vi "Main_FPGA_1_2.vi"() -> ()   [LabVIEW 2018]
uses:
  <vilib>/FPGAPlugInAG/NI 9148/niLvFpga_Open_NI 9148.vi
  <vilib>/rvi/interface/common/dynamic/niFpgaDynamicAddResources.vi
  <vilib>/FPGAPlugInAG/Dynamic/niLvFpga_Reset_Dynamic.vi
  <vilib>/FPGAPlugInAG/Dynamic/niLvFpga_Run_Dynamic.vi
  <vilib>/FPGAPlugInAG/cRIO-9082/niLvFpga_Open_cRIO-9082.vi
  <vilib>/addons/control/pid/pid.llb/PID (DBL).vi
  <vilib>/rvi/errors/niLvFpgaAdjustHostInterfaceError.vi
  <vilib>/FPGAPlugInAG/Dynamic/niLvFpga_Abort_Dynamic.vi
  <vilib>/FPGAPlugInAG/Dynamic/niLvFpga_Close_Dynamic.vi
  <vilib>/Utility/file.llb/Write Delimited Spreadsheet (string).vi
  <vilib>/rvi/interface/nirviOpenFPGA/nirviOpenFPGA.xnode
  FPGA Bitfiles/Expansion chassis.lvbitx
  Main_Mess_FPGA.vi
  <vilib>/rvi/interface/nirviMethod/nirviMethod.xnode
  FPGA Bitfiles/Main_FPGA_V3.lvbitx
  Main_FPGA.vi
  <vilib>/rvi/interface/nirviReadWriteControl/nirviReadWriteControl.xnode
  <vilib>/rvi/interface/nirviCloseFPGA/nirviCloseFPGA.xnode
  <vilib>/rvi/interface/Simulation/niFpgaSimulationCallBeginRW.vi
  <vilib>/addons/control/pid/NI_PID_pid.lvlib
  NiFpgaLv.dll
panel:
  in  "File Nmae":string
  out "Engine_Limits":refnum<vi>[](array[refnum])
  out "Pressure_Limits":refnum<vi>[](array[refnum])
  out "Pressure_Sensors":refnum<vi>[](array[refnum])
  out "Temp_Limits":refnum<vi>[](array[refnum])
  out "error out":errorcluster
  in  "Config_Save":bool
  out "Config File":path
  in  "Power_Max_Lim":dbl=100.0
  in  "Oil_P":T1={"Gain"=1.0, "offset"=0.0}
  in  "Exhaust_P":T1={"Gain"=0.5, "offset"=0.0}
  in  "Coolant-Out_P":T1={"Gain"=0.5, "offset"=0.0}
  in  "Coolant-In_P":T1={"Gain"=0.5, "offset"=0.0}
  in  "Intercooler-In_P":T1={"Gain"=1.0, "offset"=0.0}
  in  "Intercooler-Out_P":T1={"Gain"=1.0, "offset"=0.0}
  in  "Misc_P":T1={"Gain"=1.0, "offset"=0.0}
  in  "Misc_P_Lim":fxp<+/-,48,10>=5.0
  in  "Intercooler-Out_P_Lim":fxp<+/-,48,10>=3.0
  in  "Intercooler-In_P_Lim":fxp<+/-,48,10>=3.0
  in  "Intercooler_Out_Temp_lim":dbl=60.0 format="%#_13g"
  out "Intercooler_Out_T":dbl(knob) scale=0.0..100.0 scale format="%3d"
  out "Boolean 7":bool
  in  "Speed_Max_Lim":dbl=8000.0
  in  "Torque_Min_Lim":dbl=-1000.0
  in  "Torque_Max_Lim":dbl=1000.0
  out "AI0":dbl
  out "AI1":dbl
  out "AI2":dbl
  out "Mod1/CH0":fxp<+/-,32,7>
  out "Mod1/CH1":fxp<+/-,32,7>
  out "Mod1/CH2":fxp<+/-,32,7>
  out "Mod1/CH3":fxp<+/-,32,7>
  out "Intercooler-Out_P":dbl(slide) scale=0.0..10.0 scale format="%#1_6g"
  out "Misc_P":dbl(slide) scale=0.0..10.0 scale format="%#1_6g"
  out "Intercooler_In_T":dbl(knob) scale=0.0..100.0 scale format="%3d"
  out "Boolean":bool
  out "Boolean 2":bool
  out "Exhaust_T":dbl(knob) scale=0.0..1000.0 scale format="%3d"
  out "Oil_T":dbl(knob) scale=0.0..140.0 scale format="%3d"
  out "Boolean 3":bool
  out "Coolant_Outlet_T":dbl(knob) scale=0.0..120.0 scale format="%3d"
  out "Boolean 5":bool
  out "Coolant_Inlet_T":dbl(knob) scale=0.0..120.0 scale format="%3d"
  out "Boolean 4":bool
  out "Basement_T":dbl(knob) scale=0.0..60.0 scale format="%3d"
  out "Boolean 6":bool
  out "Speed Summary":dbl(knob) scale=0.0..8000.0
  out "Torque Summary":dbl(knob) scale=-500.0..1000.0
  out "Power":dbl(knob) scale=0.0..300.0
  out "Oil_P":dbl(slide) scale=0.0..10.0 scale format="%#1.1g"
  out "Exhaust_P":dbl(slide) scale=0.0..5.0 scale format="%#1_6g"
  out "Coolant-Out_P":dbl(slide) scale=0.0..5.0
  out "Intercooler-In_P":dbl(slide) scale=0.0..10.0 scale format="%2d"
  out "Coolant-In_P":dbl(slide) scale=0.0..5.0
  in  "Data_Log":bool
  in  "Coolant_Inlet_Temp_Lim":dbl=95.0 format="%#_13g"
  in  "Oil_Pres_Max_lim":fxp<+/-,48,10>=7.0
  in  "Exhaust_Pres_Lim":fxp<+/-,48,10>=3.0
  in  "CoolantOut_press_Lim":fxp<+/-,48,10>=3.0
  in  "Intercooler_In_Temp_lim":dbl=90.0 format="%#_13g"
  in  "Exhaust_Temp_Lim":dbl=730.0 format="%#_13g"
  in  "Coolant_Outlet_Temp_Lim":dbl=100.0 format="%#_13g"
  in  "Coolant In Pres_Lim":fxp<+/-,48,10>=3.0
  in  "Oil_Temp_Max_Lim":dbl=120.0 format="%#_13g"
  in  "Oil_Temp_min_Lim":dbl=20.0 format="%#_13g"
  in  "Oil_Pres_Min_lim":fxp<+/-,48,10>=1.0
  out "Saftey_Lim_error":bool
  in  "Ambient_pressure":fxp<+/-,48,10>=0.9399999999986903
  in  "Basement_Temp_Lim":dbl=2000.0 format="%#_13g"
  in  "Pres_min_spd_lim":dbl=800.0
  out "Waveform Chart - Dark":cluster{"Numeric":dbl, "Numeric":dbl}(graph)
  out "Temperature out":dbl
  in  "PID gains":T2={"proportional gain (Kc)"=1.0, "integral time (Ti, min)"=0.1, "derivative time (Td, min)"=0.0} {"derivative time (Td, min)" format="%.3f"; "integral time (Ti, min)" format="%.3f"; "proportional gain (Kc)" format="%.3f"}
  in  "Output range":cluster{"Output high":dbl, "Output low":dbl}={"Output high"=10.0, "Output low"=0.0} {"Output low" format="%.2f"; "Output high" format="%.2f"}
  in  "Temperature PID":bool=TRUE
  in  "Temperature":dbl(slide) scale=0.0..100.0
  in  "Stop":bool
  # "Engine Safety Limits"
  # "Pressure Safety Limits"
  # "Temp Safety Limits"
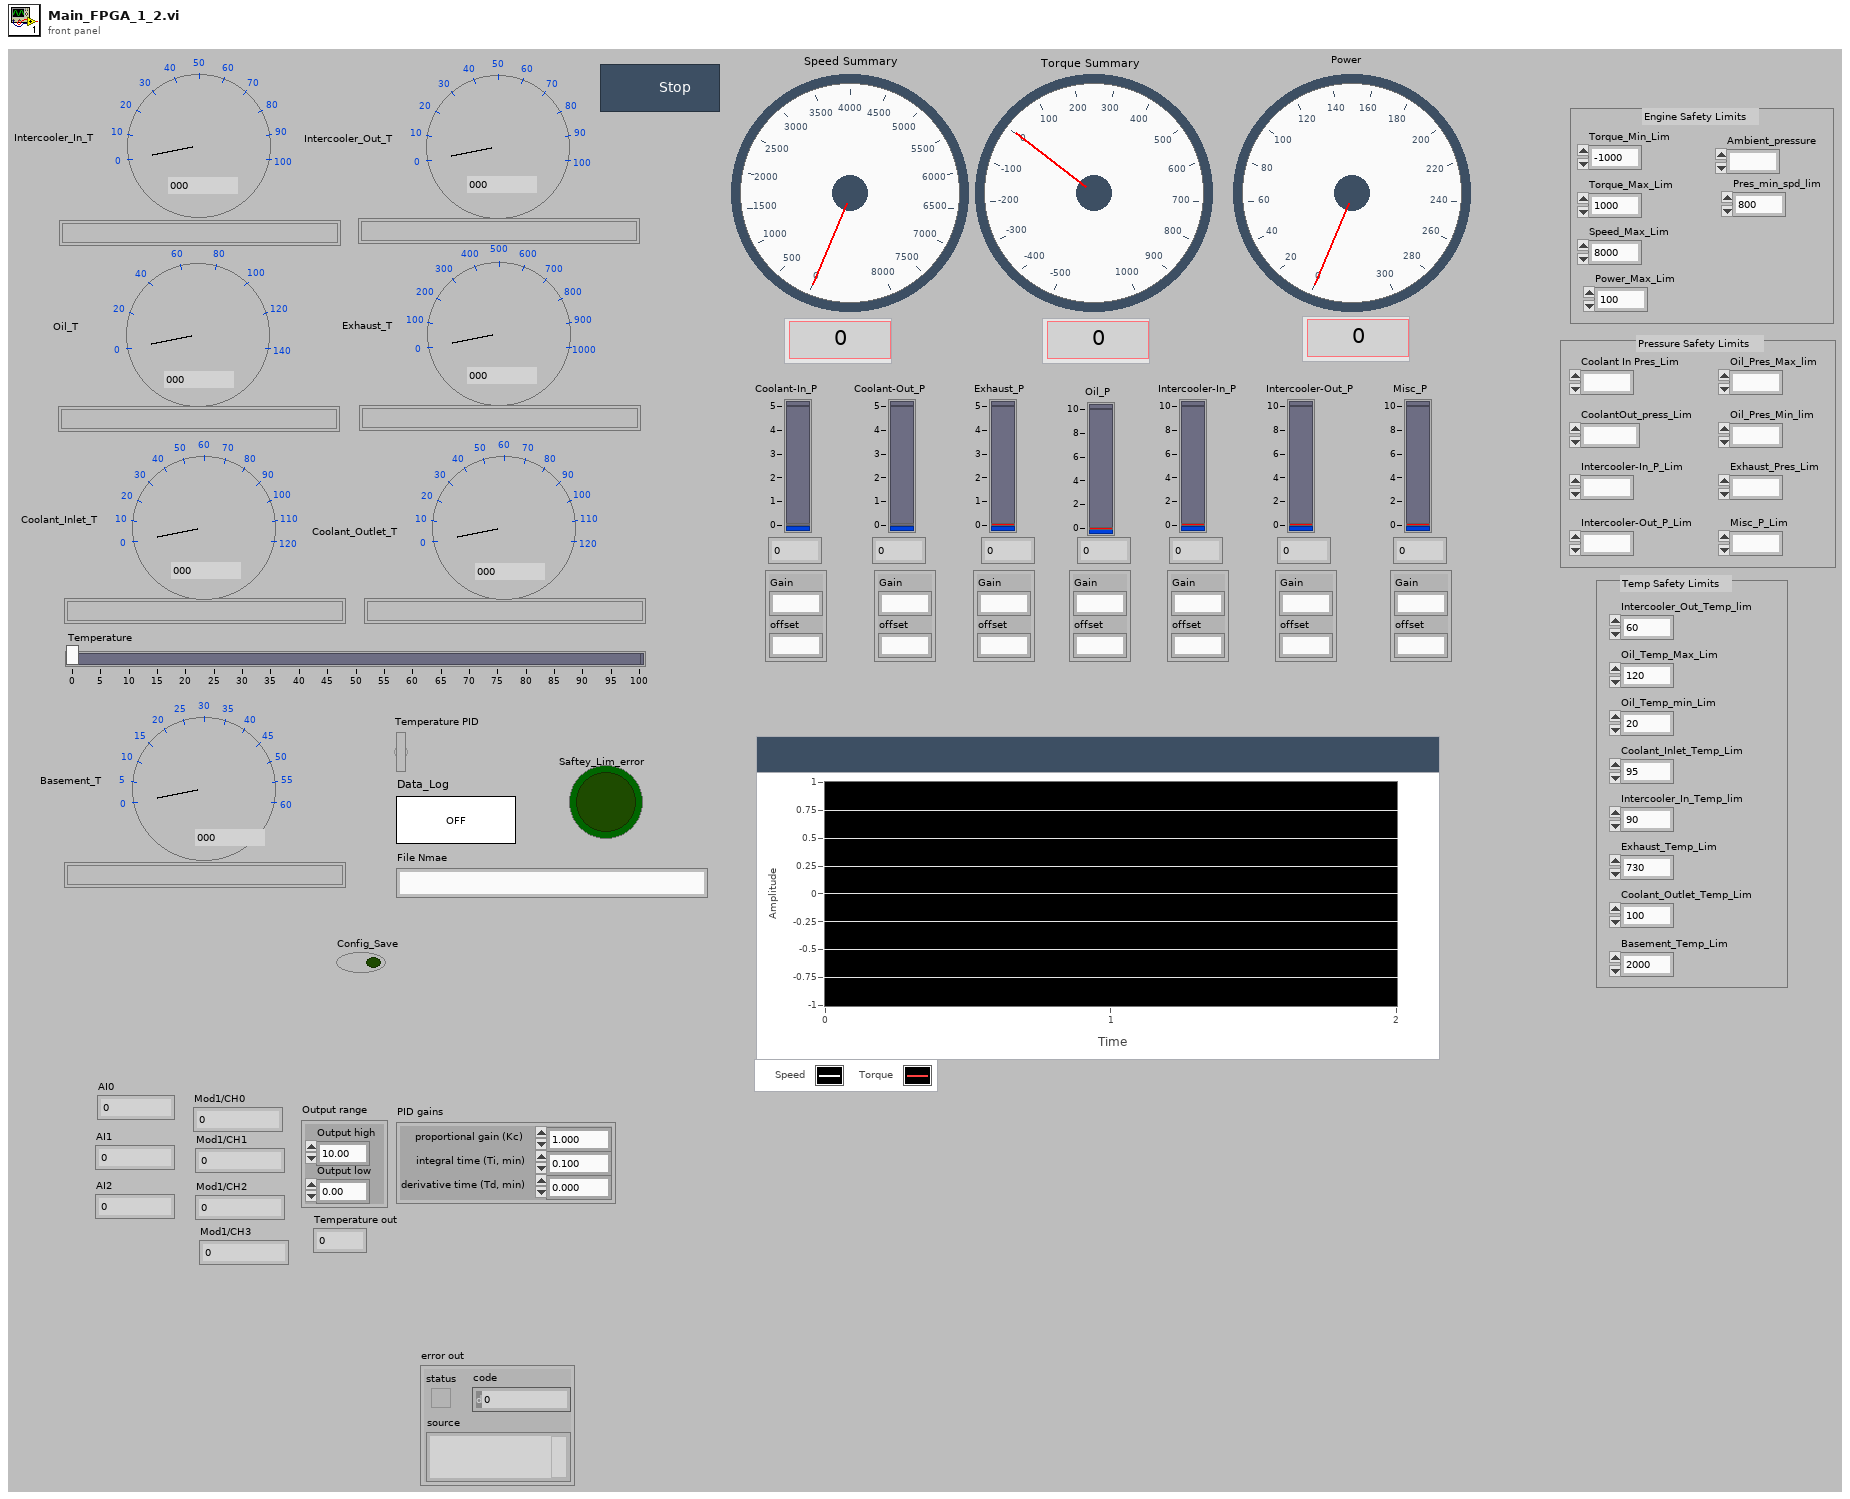
[diagram p1: front panel]
types:
  T1 = cluster{"Gain":fxp<+/-,24,5>, "offset":fxp<+/-,24,5>}
  T2 = cluster{"proportional gain (Kc)":dbl, "integral time (Ti, min)":dbl, "derivative time (Td, min)":dbl}
  T3 = enum32{"Invalid", "Standard", "Closed", "Hidden", "Minimized", "Maximized"}
  T4 = enum32{"invalid app kind", "Development System", "Run Time System", "Student Edition", "Embedded LabVIEW", "Evaluation", "Custom"}
  T5 = cluster{"Core":cluster{"Current VI Reference":refnum<vi>, "Close Panel on Exit?":bool}, "Intercooler_In_T":refnum<vi>, "Coolant_Inlet_T":refnum<vi>, "Coolant_Outlet_T":refnum<vi>, "Basement_T":refnum<vi>, "Exhaust_T":refnum<vi>, "Oil_T":refnum<vi>, "Intercooler_Out_T":refnum<vi>, "ExpansionChassFPGA":refnum<k20>}
  T6 = cluster{"Current VI Reference":refnum<vi>, "Close Panel on Exit?":bool}
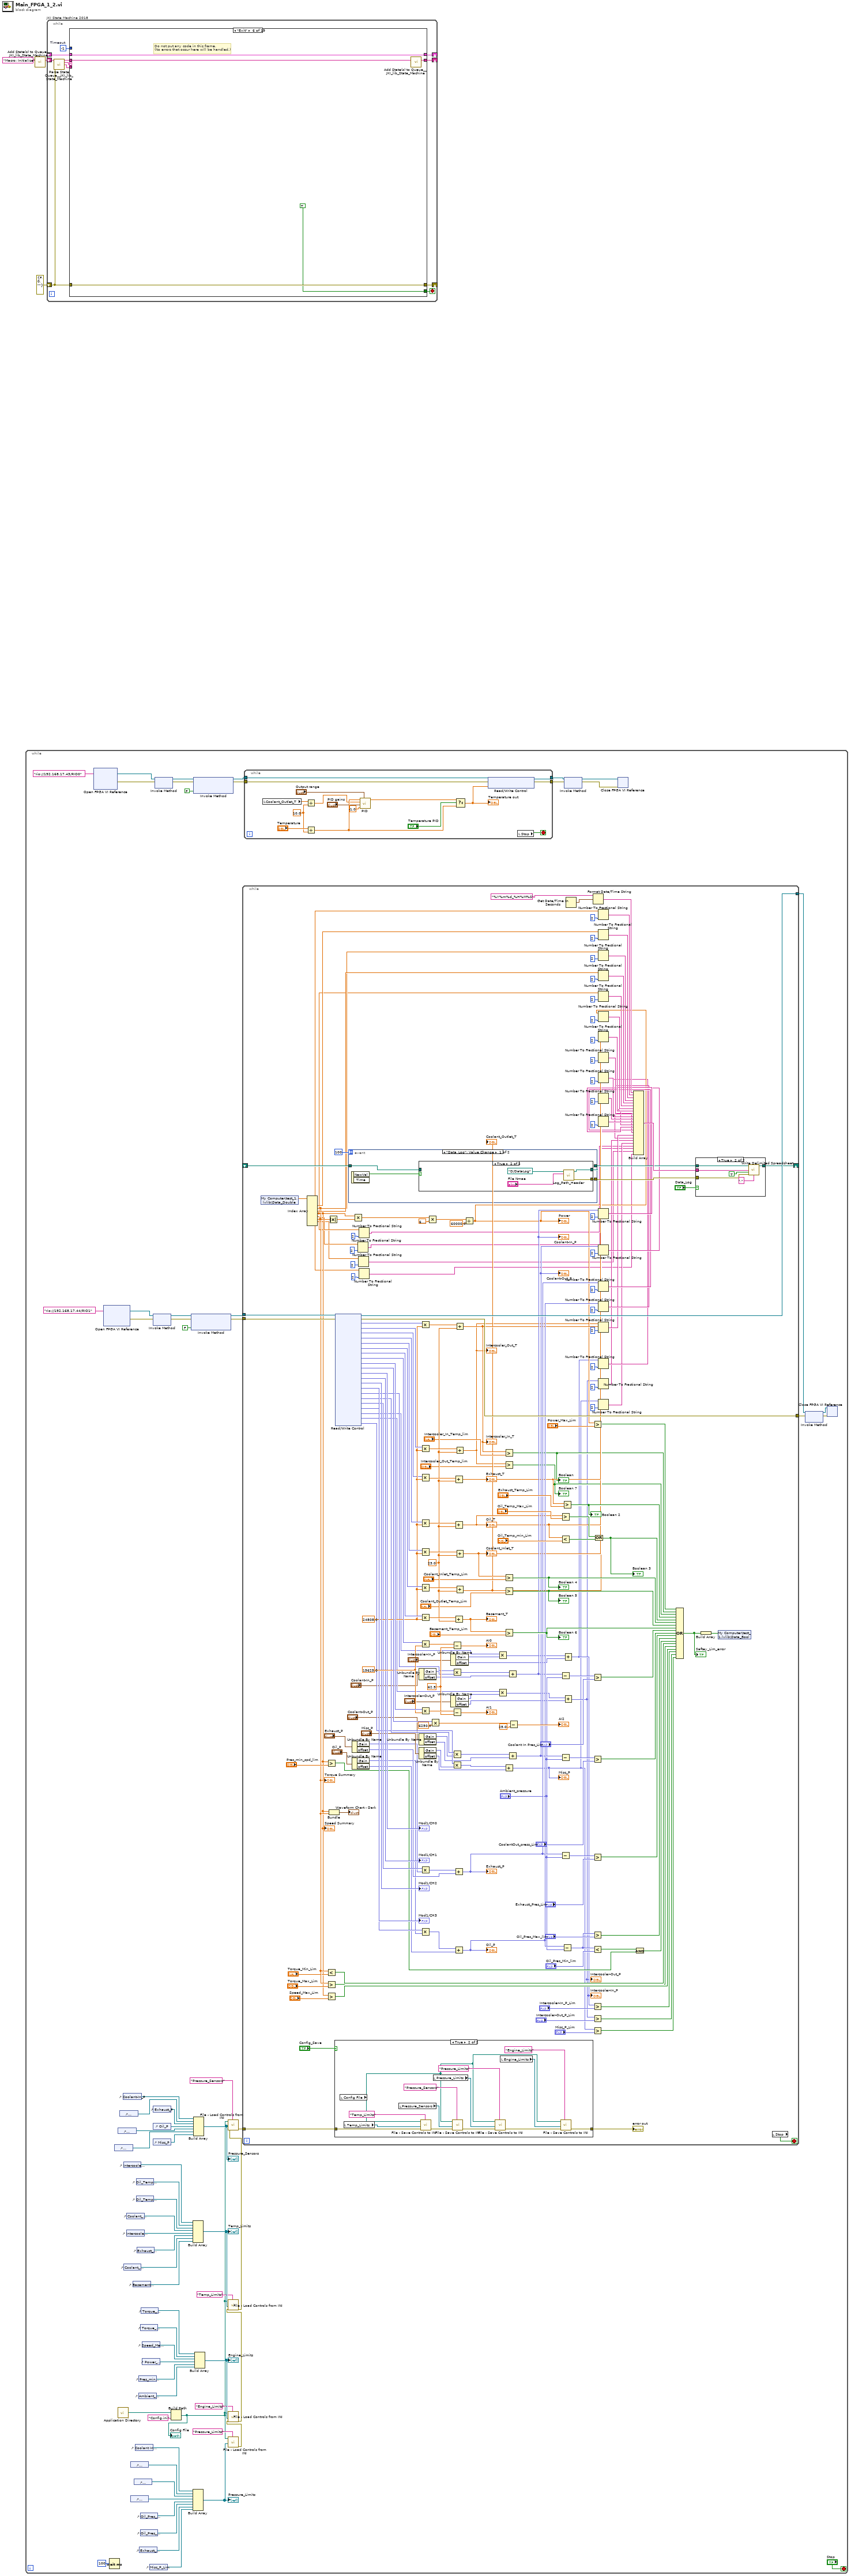
[diagram p0: block diagram]
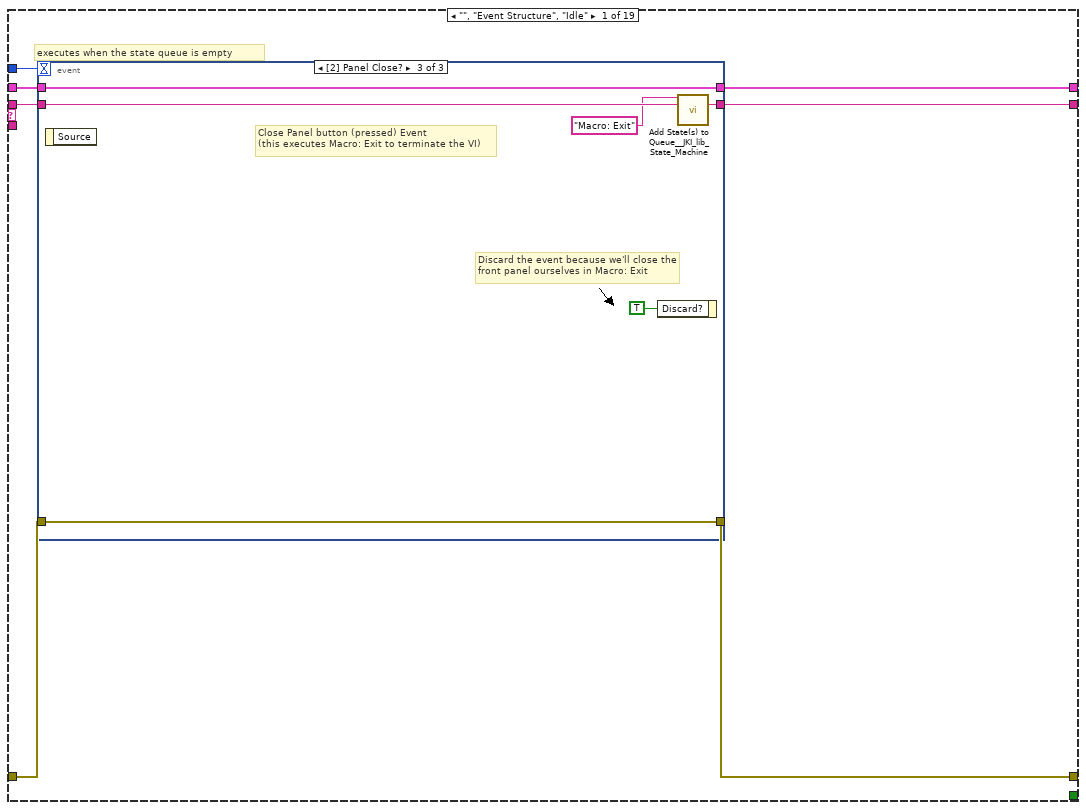
[diagram p2: hidden frame]
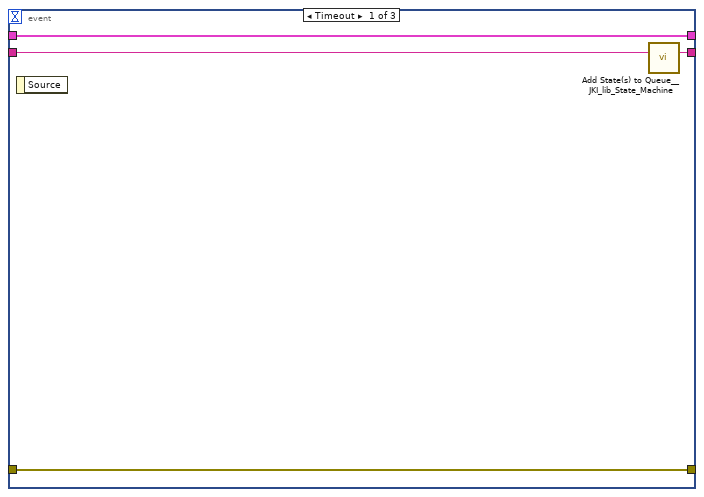
[diagram p3: hidden frame]
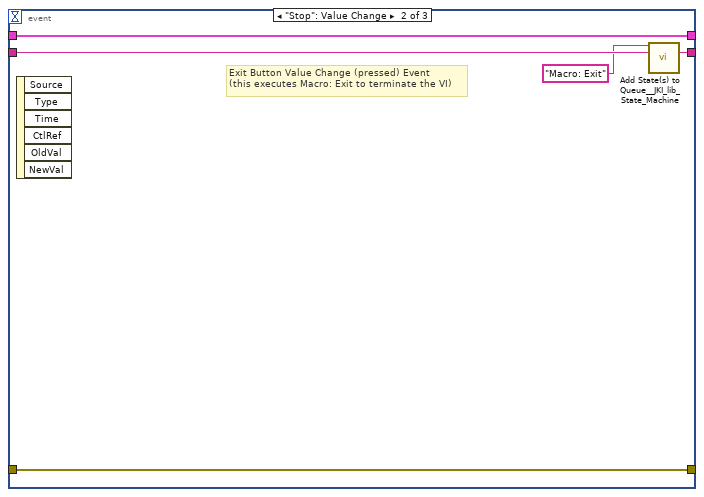
[diagram p4: hidden frame]
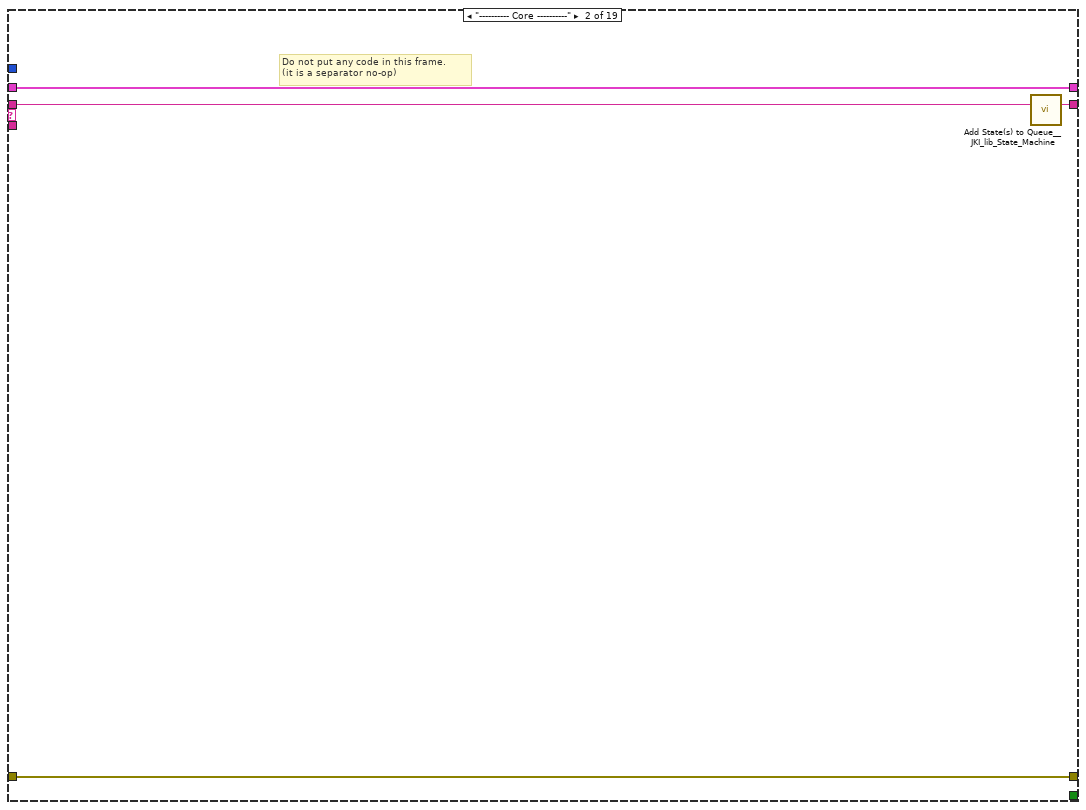
[diagram p5: hidden frame]
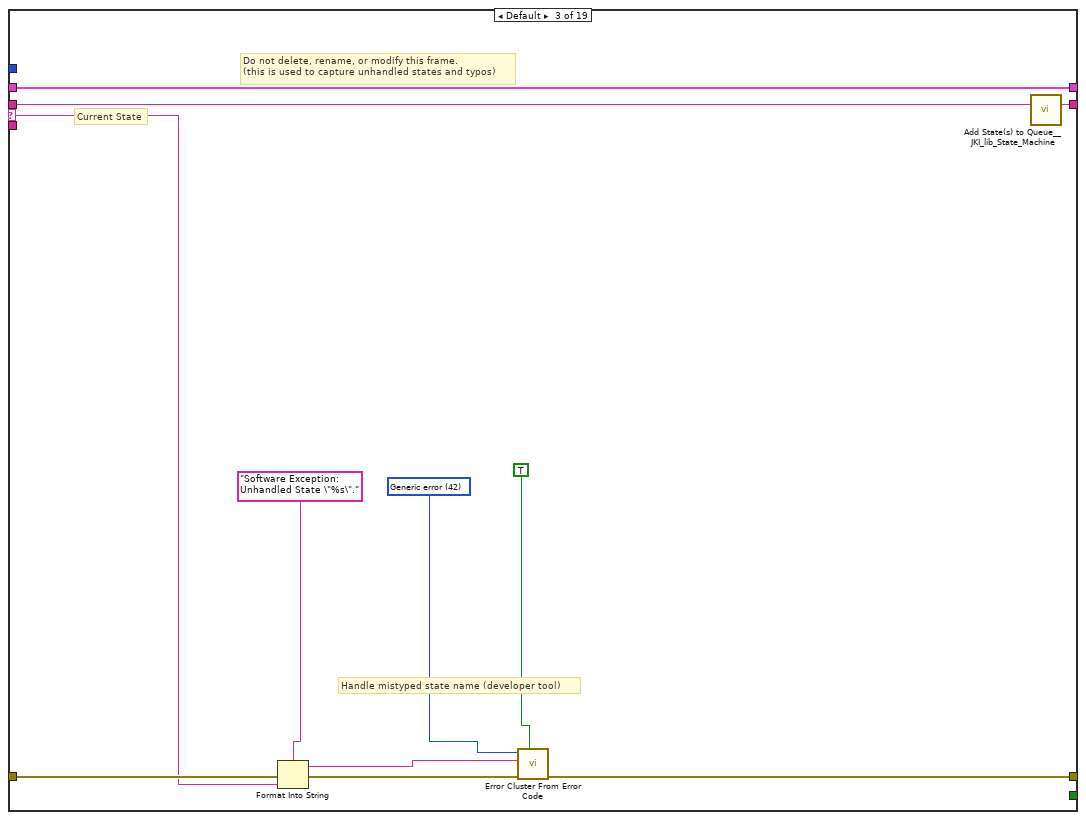
[diagram p6: hidden frame]
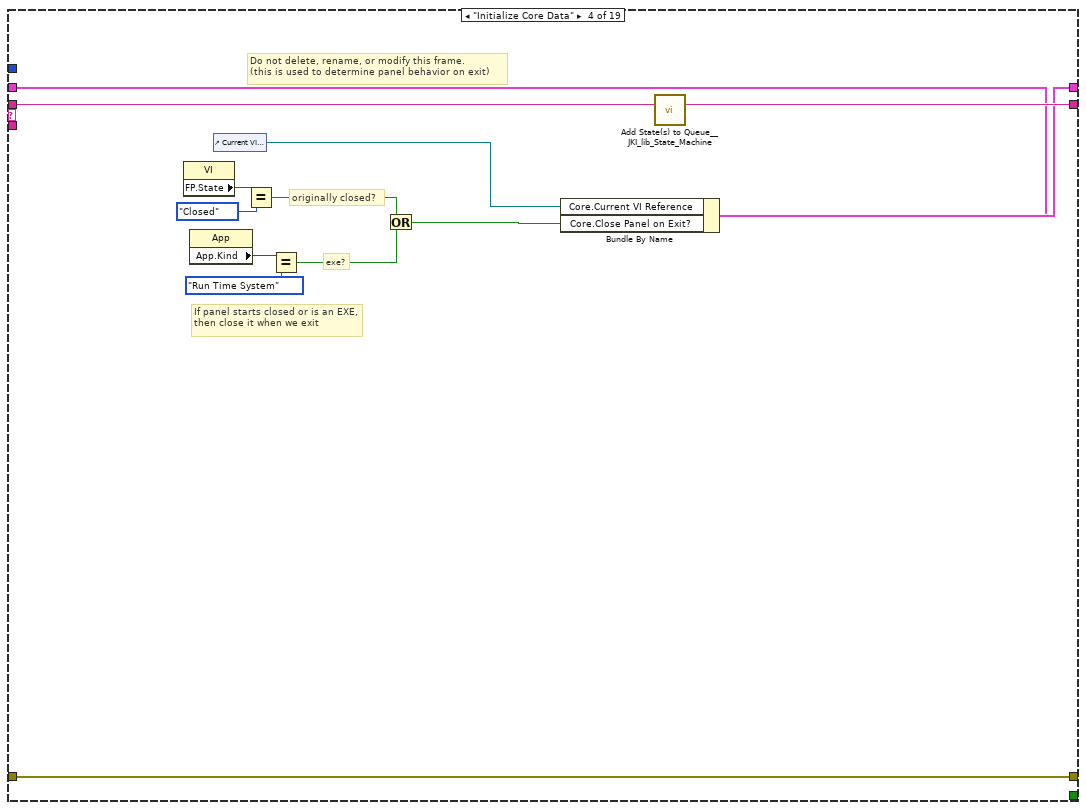
[diagram p7: hidden frame]
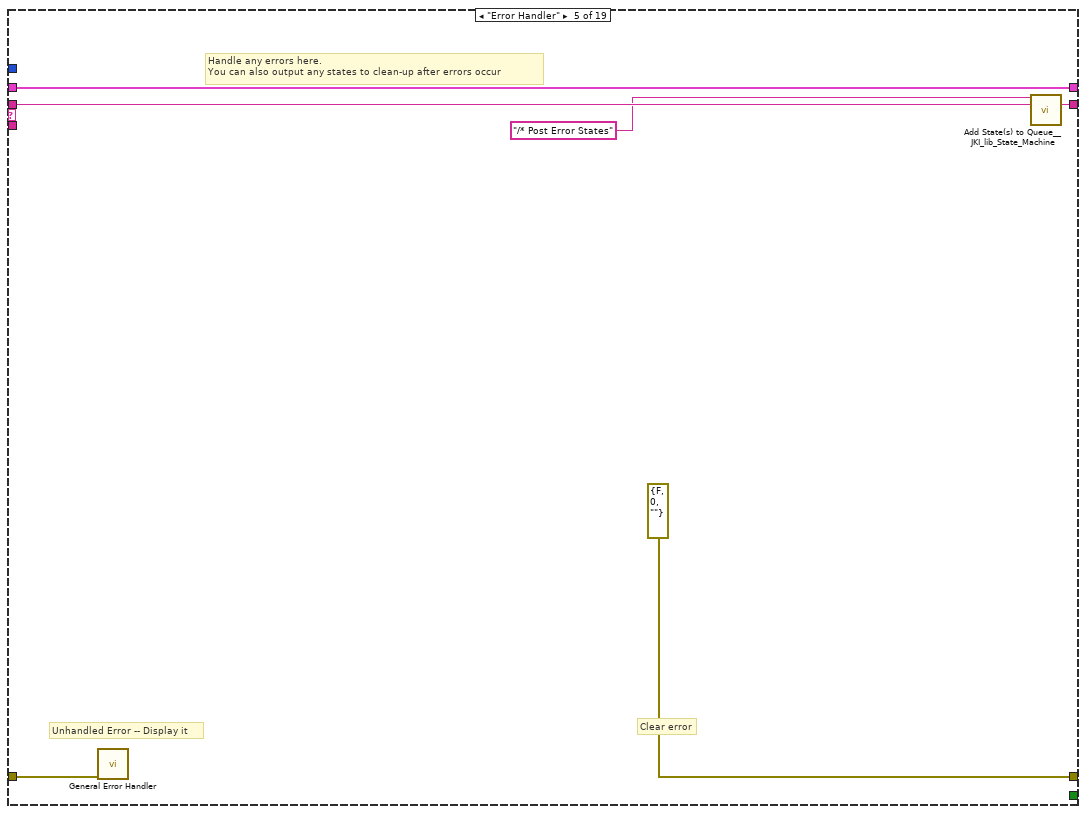
[diagram p8: hidden frame]
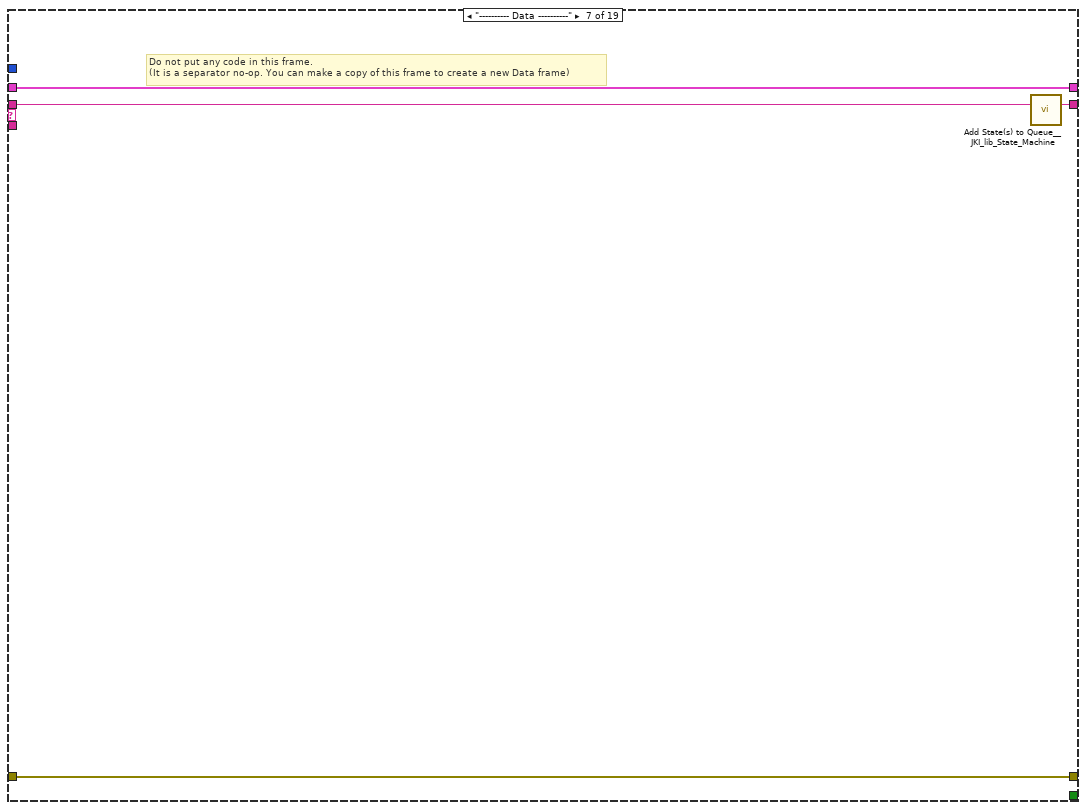
[diagram p9: hidden frame]
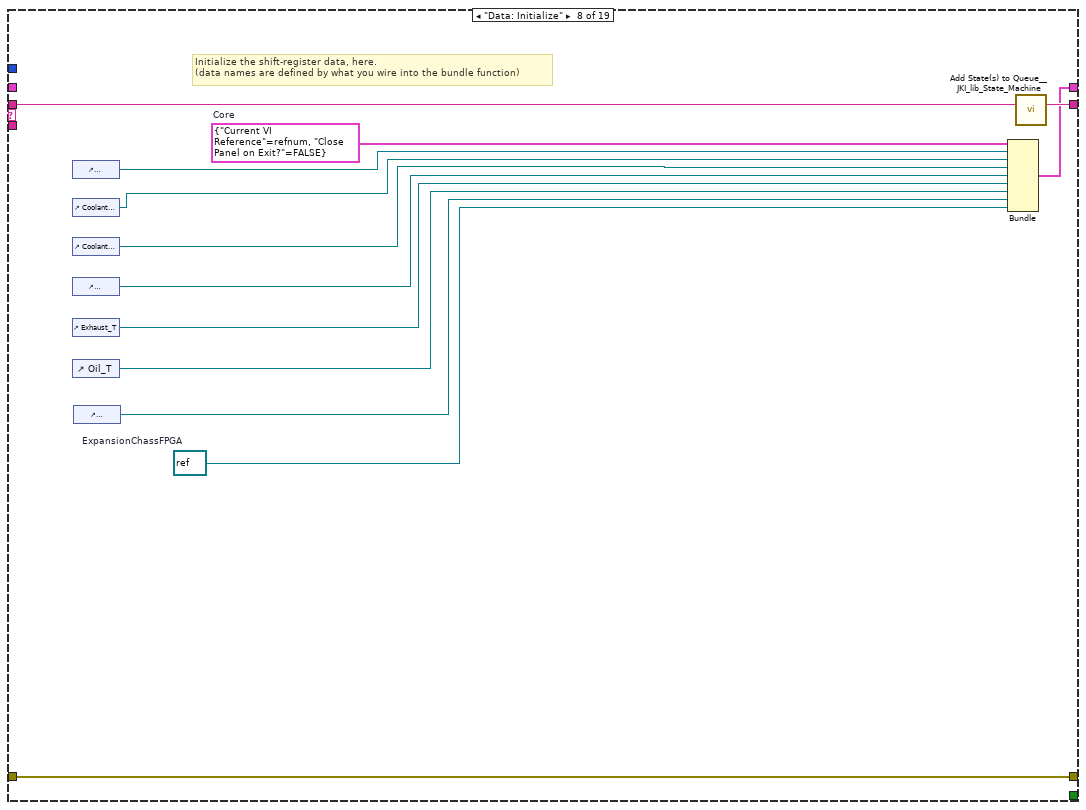
[diagram p10: hidden frame]
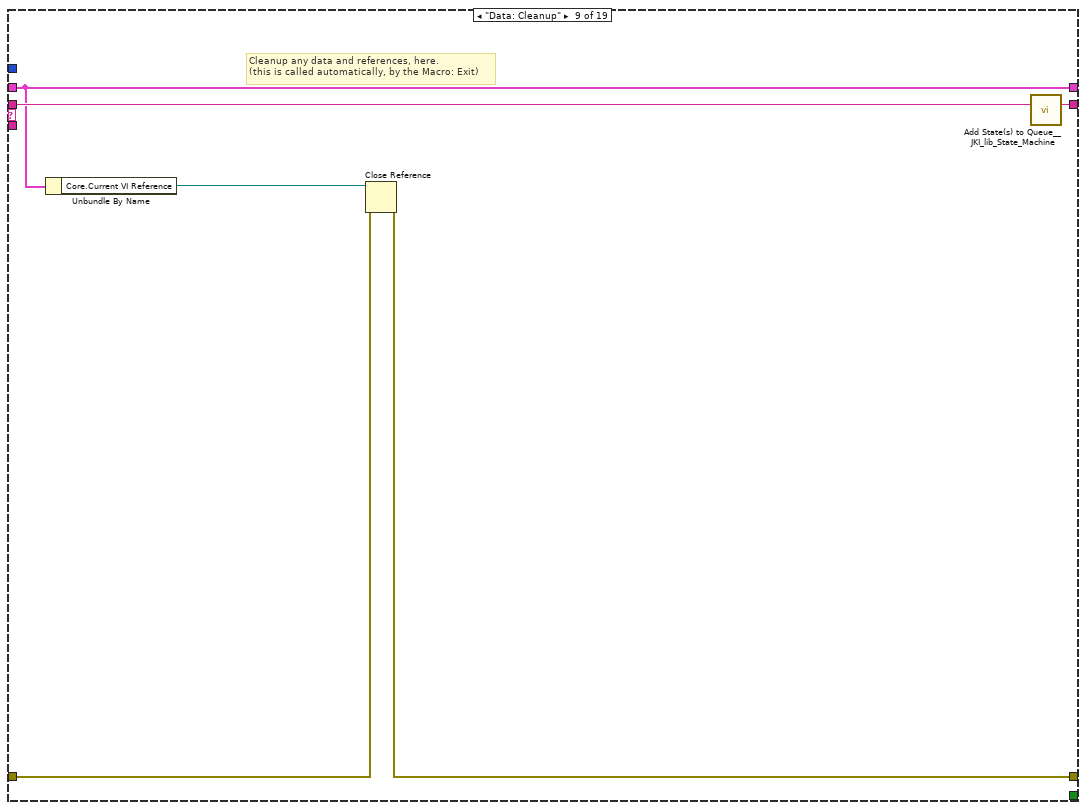
[diagram p11: hidden frame]
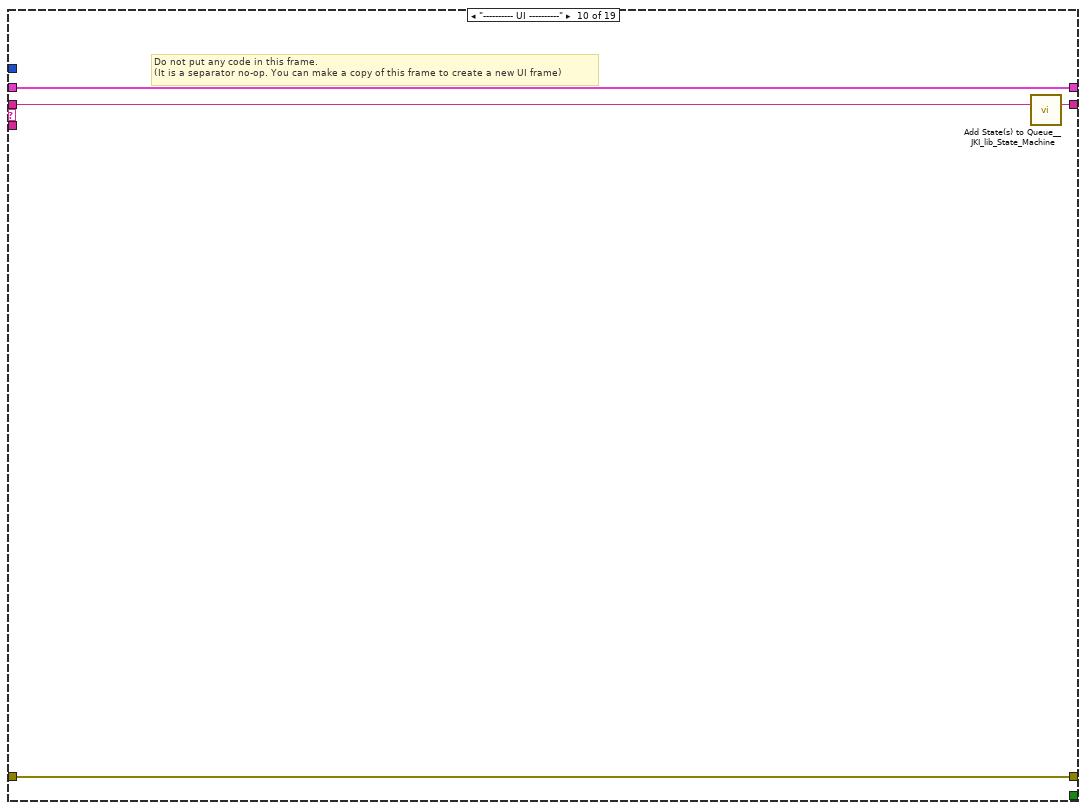
[diagram p12: hidden frame]
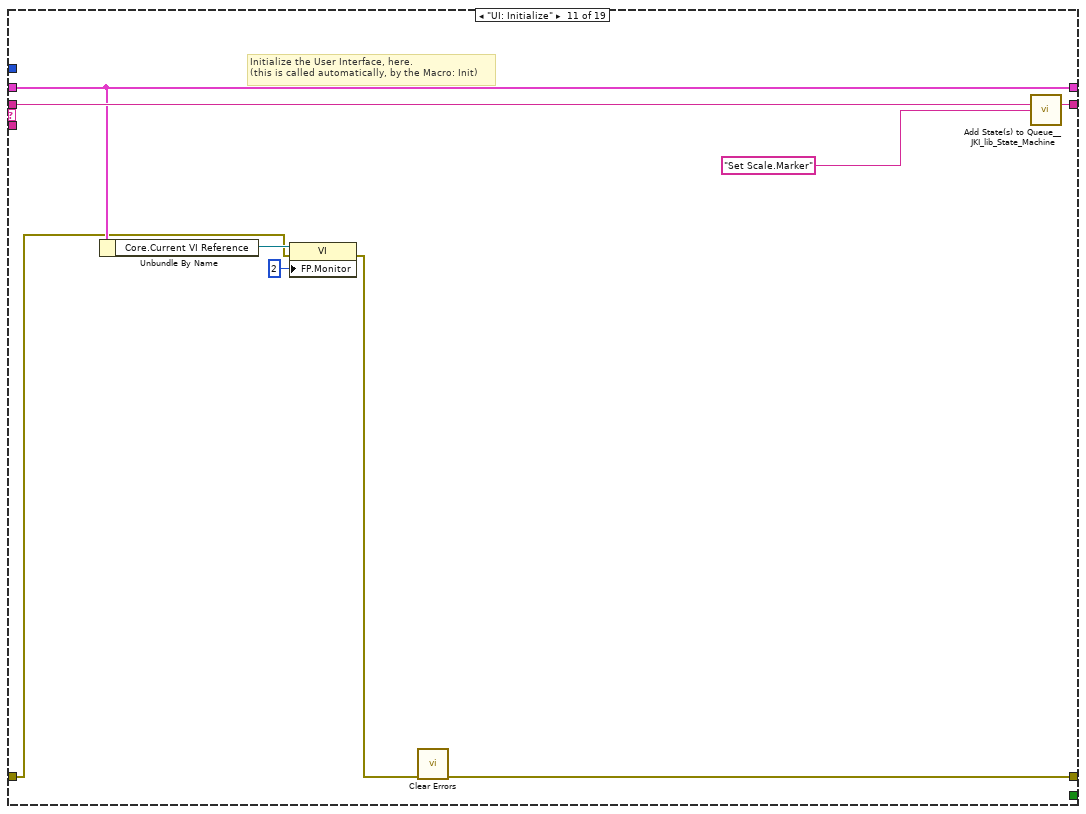
[diagram p13: hidden frame]
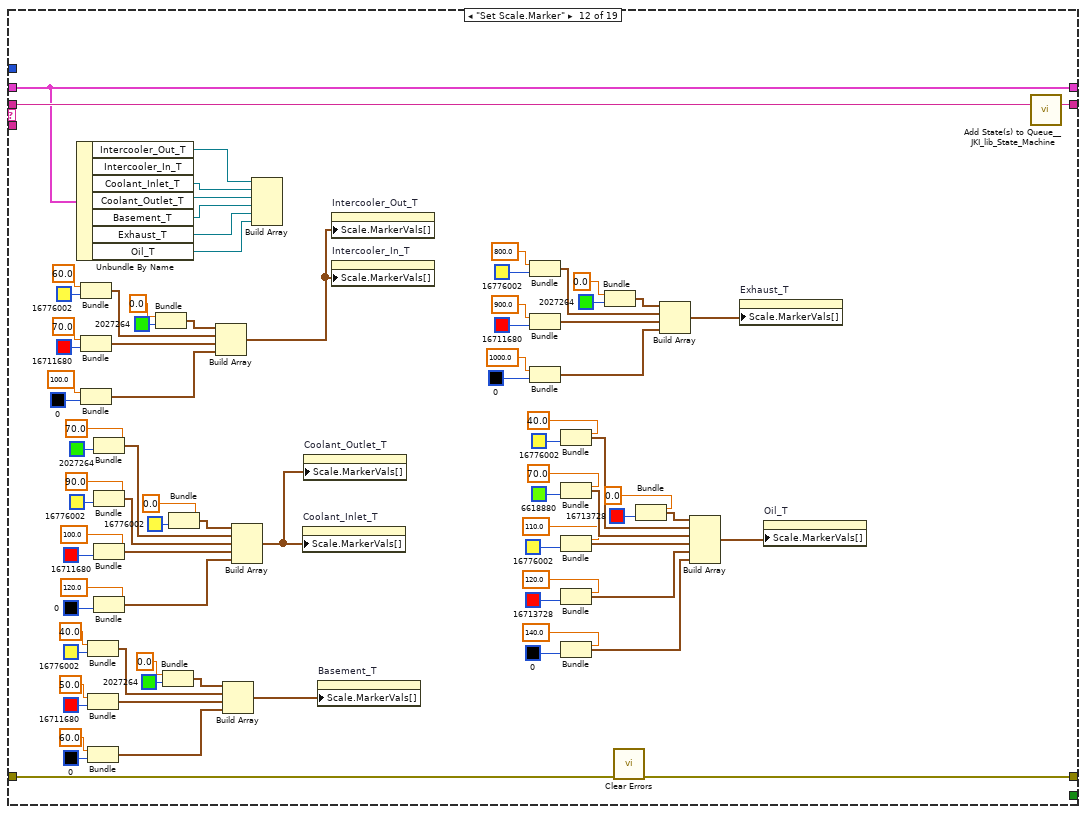
[diagram p14: hidden frame]
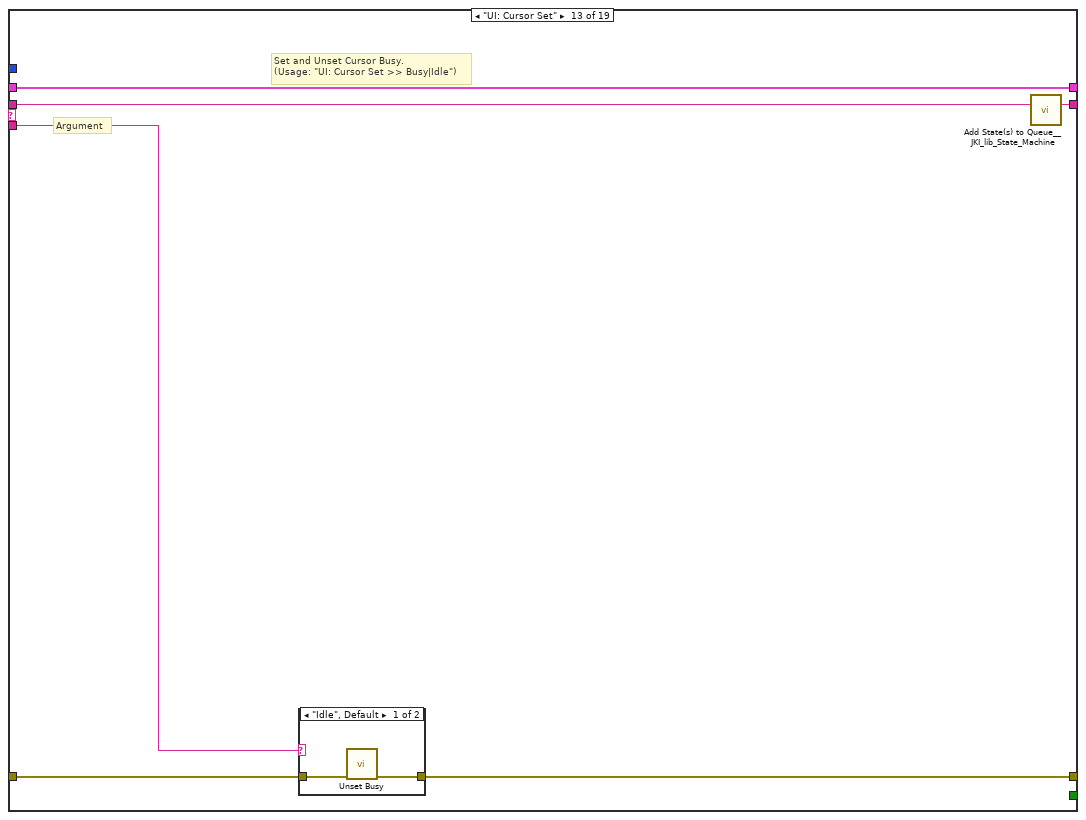
[diagram p15: hidden frame]
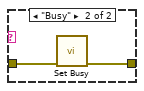
[diagram p16: hidden frame]
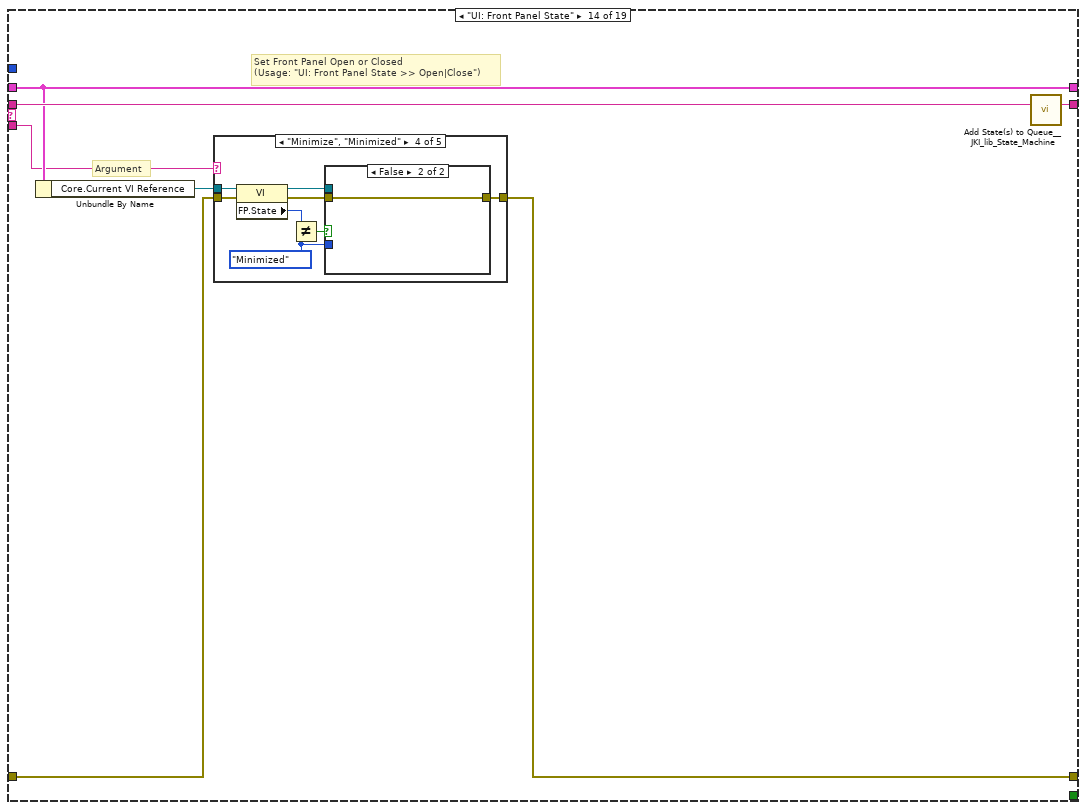
[diagram p17: hidden frame]
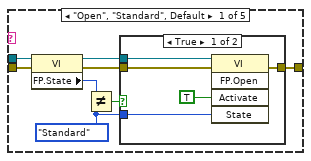
[diagram p18: hidden frame]
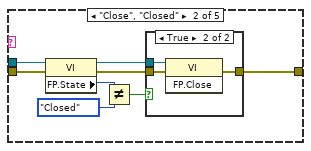
[diagram p20: hidden frame]
diagram:
  n1 = while {
    stop <- "Stop" stop-if-true
    n2 = xnode "Open FPGA VI Reference"("resource name"=tag "rio://192.168.17.43/RIO0") -> ("FPGA VI Reference Out"=w65:refnum<k20>, "error out"=w64:errorcluster)  [unwired: 1 in]
    n3 = xnode "Open FPGA VI Reference"("resource name"=tag "rio://192.168.17.44/RIO1") -> ("FPGA VI Reference Out"=w68:refnum<k20>, "error out"=w72:errorcluster)  [unwired: 1 in]
    n4 = Wait (ms)(milliseconds to wait=u32 100) -> ()  [unwired: 1 out]
    n5 = control-ref of="Intercooler-Out_P"() -> (w44:refnum<vi>)
    n6 = control-ref of="Intercooler-In_P"() -> (w45:refnum<vi>)
    n7 = call <vilib>:"Application Directory.vi"() -> ("Application Directory"=w8:path)
    n8 = control-ref of="Coolant-Out_P"() -> (w48:refnum<vi>)
    n9 = control-ref of="Coolant-In_P"() -> (w49:refnum<vi>)
    n10 = control-ref of="Intercooler_Out_Temp_lim"() -> (w28:refnum<vi>)
    n11 = control-ref of="Coolant_Outlet_Temp_Lim"() -> (w22:refnum<vi>)
    n12 = control-ref of="Coolant_Inlet_Temp_Lim"() -> (w25:refnum<vi>)
    n13 = control-ref of="Intercooler_In_Temp_lim"() -> (w24:refnum<vi>)
    n14 = control-ref of="CoolantOut_press_Lim"() -> (w35:refnum<vi>)
    n15 = control-ref of="Intercooler-Out_P_Lim"() -> (w33:refnum<vi>)
    n16 = control-ref of="Basement_Temp_Lim"() -> (w21:refnum<vi>)
    n17 = control-ref of="Intercooler-In_P_Lim"() -> (w34:refnum<vi>)
    n18 = control-ref of="Coolant In Pres_Lim"() -> (w36:refnum<vi>)
    n19 = control-ref of="Oil_Temp_Max_Lim"() -> (w27:refnum<vi>)
    n20 = control-ref of="Oil_Temp_min_Lim"() -> (w26:refnum<vi>)
    n21 = control-ref of="Exhaust_Temp_Lim"() -> (w23:refnum<vi>)
    n22 = control-ref of="Pres_min_spd_lim"() -> (w38:refnum<vi>)
    n23 = control-ref of="Ambient_pressure"() -> (w37:refnum<vi>)
    n24 = control-ref of="Exhaust_Pres_Lim"() -> (w30:refnum<vi>)
    n25 = control-ref of="Torque_Max_Lim"() -> (w41:refnum<vi>)
    n26 = control-ref of="Oil_Pres_Max_lim"() -> (w32:refnum<vi>)
    n27 = control-ref of="Oil_Pres_Min_lim"() -> (w31:refnum<vi>)
    n28 = control-ref of="Torque_Min_Lim"() -> (w42:refnum<vi>)
    n29 = control-ref of="Speed_Max_Lim"() -> (w40:refnum<vi>)
    n30 = control-ref of="Power_Max_Lim"() -> (w39:refnum<vi>)
    n31 = control-ref of="Misc_P_Lim"() -> (w29:refnum<vi>)
    n32 = xnode "Invoke Method"("FPGA VI Reference In"=w68, "error in"=w72) -> ("FPGA VI Reference Out"=w69:refnum<k20>, "error out"=w71:errorcluster)
    n33 = control-ref of="Exhaust_P"() -> (w47:refnum<vi>)
    n34 = control-ref of="Oil_P"() -> (w46:refnum<vi>)
    n35 = control-ref of="Misc_P"() -> (w43:refnum<vi>)
    n36 = xnode "Invoke Method"("FPGA VI Reference In"=w65, "error in"=w64) -> ("FPGA VI Reference Out"=w63:refnum<k20>, "error out"=w62:errorcluster)
    n37 = Build Path(base path=w8, name or relative path="Config.ini") -> (appended path=w6:path)
    "Config File" <- w6
    n38 = xnode "Invoke Method"("FPGA VI Reference In"=w69, "error in"=w71, "Wait Until Done (F)"=FALSE) -> ("FPGA VI Reference Out"=w53:refnum<k20>, "error out"=w52:errorcluster)
    n39 = Build Array(w28, w27, w26, w25, w24, w23, w22, w21) -> (w18:refnum<vi>[])
    "Temp_Limits" <- w18
    n40 = Build Array(w36, w35, w34, w33, w32, w31, w30, w29) -> (w13:refnum<vi>[])
    "Pressure_Limits" <- w13
    n41 = xnode "Invoke Method"("FPGA VI Reference In"=w63, "error in"=w62, "Wait Until Done (F)"=FALSE) -> ("FPGA VI Reference Out"=w60:refnum<k20>, "error out"=w59:errorcluster)
    n42 = Build Array(w49, w48, w47, w46, w45, w44, w43) -> (w20:refnum<vi>[])
    "Pressure_Sensors" <- w20
    n43 = Build Array(w42, w41, w40, w39, w38, w37) -> (w16:refnum<vi>[])
    "Engine_Limits" <- w16
    n44 = call "File - Load Controls from INI.vi"("Section"="Pressure_Limits", "Array of References"=w13, "INI File"=w6) -> ("error out"=w9:errorcluster)  [unwired: 8 in]
    n45 = call "File - Load Controls from INI.vi"("Section"="Engine_Limits", "error in (no error)"=w9, "Array of References"=w16, "INI File"=w6) -> ("error out"=w10:errorcluster)  [unwired: 7 in]
    n46 = call "File - Load Controls from INI.vi"("Section"="Temp_Limits", "error in (no error)"=w10, "Array of References"=w18, "INI File"=w6) -> ("error out"=w11:errorcluster)  [unwired: 7 in]
    n47 = call "File - Load Controls from INI.vi"("Section"="Pressure_Sensors", "error in (no error)"=w11, "Array of References"=w20, "INI File"=w6) -> ("error out"=w12:errorcluster)  [unwired: 7 in]
    n48 = while {
      tunnel: w53 -> [w287]
      tunnel: [w286] -> w51
      tunnel: [w285] -> w50
      tunnel: w52 -> [w284]
      shift-right: [w225] -> _
      shift-left: _ -> [w224]
      tunnel: w12 -> [w86]
      stop <- w282 stop-if-true
      w269 = 62.5 ("y")
      w272 = 15625.0
      w251 = 23.0 ("y")
      w252 = 24808.0 ("y")
      n49 = shared-variable "My Computer\\test_1.lvlib\\Data_Double"() -> (w171:dbl[])  [unwired: 1 in, 1 out]
      n50 = Index Array(array=w171) -> (element #1=w170:dbl, element #2=w168:dbl, element #3=w146:dbl, element #4=w167:dbl, element #5=w142:dbl, element #6=w81:dbl, element #7=w80:dbl, element #8=w79:dbl, element #9=w78:dbl)  [unwired: 9 in]
      "Speed Summary" <- w142
      "Torque Summary" <- w146
      n51 = Greater?(x=w142, y="Pres_min_spd_lim") -> (0:w179:bool)
      n52 = Less?(x=w146, y="Torque_Min_Lim") -> (x < y?=w144:bool)
      n53 = Greater?(x=w146, y="Torque_Max_Lim") -> (0:w143:bool)
      n54 = Greater?(x=w142, y="Speed_Max_Lim") -> (0:w140:bool)
      n55 = Absolute Value(x=w146) -> (abs(x)=w239:dbl)
      n56 = Bundle("Numeric"=w142, "Numeric"=w146) -> (→"Waveform Chart - Dark":cluster{"Numeric":dbl, "Numeric":dbl})  [unwired: 1 in]
      n57 = case shown="True" "Config_Save" {
        tunnel: [w288 w290] -> w87
        tunnel: w86 -> [w288 w289]
        frame False {
        }
        frame True {
          n58 = local read "Config File"() -> (w293:path)
          n59 = local read "Temp_Limits"() -> (w302:refnum<vi>[])
          n60 = local read "Pressure_Sensors"() -> (w299:refnum<vi>[])
          n61 = call "File - Save Controls to INI.vi"("Section"="Temp_Limits", "error in (no error)"=w289, "Array of References"=w302, "INI File"=w293) -> ("error out"=w301:errorcluster)  [unwired: 7 in]
          n62 = local read "Pressure_Limits"() -> (w295:refnum<vi>[])
          n63 = call "File - Save Controls to INI.vi"("Section"="Pressure_Sensors", "error in (no error)"=w301, "Array of References"=w299, "INI File"=w293) -> ("error out"=w297:errorcluster)  [unwired: 7 in]
          n64 = call "File - Save Controls to INI.vi"("Section"="Pressure_Limits", "error in (no error)"=w297, "Array of References"=w295, "INI File"=w293) -> ("error out"=w294:errorcluster)  [unwired: 7 in]
          n65 = local read "Engine_Limits"() -> (w291:refnum<vi>[])
          n66 = call "File - Save Controls to INI.vi"("Section"="Engine_Limits", "error in (no error)"=w294, "Array of References"=w291, "INI File"=w293) -> ("error out"=w290:errorcluster)  [unwired: 7 in]
        }
      }
      "error out" <- w87
      n67 = xnode "Read/Write Control"("FPGA VI Reference In"=w287, "error in"=w284) -> ("FPGA VI Reference Out"=w286:refnum<k20>, "error out"=w285:errorcluster, "Mod7/TC0"=w257:fxp<+/-,24,-2>, "Mod7/TC1"=w258:fxp<+/-,24,-2>, "Mod7/TC2"=w238:fxp<+/-,24,-2>, "Mod7/TC3"=w256:fxp<+/-,24,-2>, "Mod7/TC4"=w259:fxp<+/-,24,-2>, "Mod7/TC5"=w255:fxp<+/-,24,-2>, "Mod7/TC6"=w254:fxp<+/-,24,-2>, "Mod4/AI0"=w277:fxp<+/-,24,-4>, "Mod4/AI1"=w274:fxp<+/-,24,-4>, "Mod4/AI2"=w273:fxp<+/-,24,-4>, "Mod1/CH0"=→"Mod1/CH0":fxp<+/-,32,7>, "Mod1/CH1"=→"Mod1/CH1":fxp<+/-,32,7>, "Mod1/CH2"=→"Mod1/CH2":fxp<+/-,32,7>, "Mod1/CH3"=→"Mod1/CH3":fxp<+/-,32,7>, "Mod2/AI0"=w231:fxp<+/-,24,5>, "Mod2/AI1"=w230:fxp<+/-,24,5>, "Mod2/AI2"=w234:fxp<+/-,24,5>, "Mod2/AI3"=w237:fxp<+/-,24,5>, "Mod2/AI4"=w138:fxp<+/-,24,5>, "Mod2/AI5"=w135:fxp<+/-,24,5>, "Mod2/AI6"=w133:fxp<+/-,24,5>)
      n68 = event shown="[0] \"Data_Log\": Value Change" {
        selector: _ -> [_ _]
        dyn-events: _ -> [_ _]
        timeout: 100 -> [_ _]
        tunnel: [w306 _] -> w227
        tunnel: [w305 w312] -> w226
        tunnel: w224 -> [w303 w312]
        event "Data_Log": Value Change {
          n69 = event-data() -> ("NewVal"=w304:bool)  [unwired: 1 in, 1 out]
          n70 = case shown="True" w304 {
            tunnel: [_ w310] -> w306
            tunnel: [w307 w309] -> w305
            tunnel: w303 -> [w307 _]
            frame False {
            }
            frame True {
              n71 = call "Log_Path_Header.vi"("File Name"="File Nmae", "start path"=path "D:/DataLog") -> ("error out"=w310:errorcluster, "path"=w309:path)  [unwired: 8 in]
            }
          }
        }
        event Timeout {
          n72 = event-data() -> ()  [unwired: 1 in, 3 out]
        }
      }
      n73 = Unbundle By Name("Exhaust_P") -> ("Gain"=w108:fxp<+/-,24,5>, "offset"=w107:fxp<+/-,24,5>)
      n74 = Unbundle By Name("Oil_P") -> ("Gain"=w105:fxp<+/-,24,5>, "offset"=w104:fxp<+/-,24,5>)
      n75 = Multiply(x=w142, y=w239) -> (x*y=w240:dbl)
      n76 = Number To Fractional String(number=w80, precision (6)=i16 2) -> (F-format string=w76:string)  [unwired: 2 in]
      n77 = Number To Fractional String(number=w79, precision (6)=i16 2) -> (F-format string=w75:string)  [unwired: 2 in]
      n78 = Number To Fractional String(number=w81, precision (6)=i16 2) -> (F-format string=w77:string)  [unwired: 2 in]
      n79 = Number To Fractional String(number=w78, precision (6)=i16 2) -> (F-format string=w74:string)  [unwired: 2 in]
      n80 = Unbundle By Name("Coolant-In_P") -> ("Gain"=w114:fxp<+/-,24,5>, "offset"=w113:fxp<+/-,24,5>)
      n81 = Unbundle By Name("Coolant-Out_P") -> ("Gain"=w111:fxp<+/-,24,5>, "offset"=w110:fxp<+/-,24,5>)
      n82 = Unbundle By Name("Misc_P") -> ("Gain"=w123:fxp<+/-,24,5>, "offset"=w122:fxp<+/-,24,5>)
      n83 = Multiply(x=w257, y=w252) -> (x*y=w281:dbl)
      n84 = Multiply(x=w258, y=w252) -> (x*y=w280:dbl)
      n85 = Multiply(x=w238, y=w252) -> (x*y=w283:dbl)
      n86 = Multiply(x=w256, y=w252) -> (x*y=w279:dbl)
      n87 = Multiply(x=w259, y=w252) -> (x*y=w260:dbl)
      n88 = Multiply(x=w255, y=w252) -> (x*y=w278:dbl)
      n89 = Multiply(x=w254, y=w252) -> (x*y=w253:dbl)
      n90 = Multiply(x=w277, y=w272) -> (x*y=w276:dbl)
      n91 = Multiply(x=w274, y=w272) -> (x*y=w271:dbl)
      n92 = Multiply(x=w234, y=w108) -> (x*y=w235:fxp<+/-,48,10>)
      n93 = Multiply(x=w237, y=w105) -> (x*y=w236:fxp<+/-,48,10>)
      n94 = Multiply(x=w240, y=6.283185307179586) -> (x*y=w241:dbl)
      n95 = Multiply(x=w273, y=6250.0) -> (x*y=w270:dbl)
      n96 = Unbundle By Name("Intercooler-In_P") -> ("Gain"=w117:fxp<+/-,24,5>, "offset"=w116:fxp<+/-,24,5>)
      n97 = Unbundle By Name("Intercooler-Out_P") -> ("Gain"=w120:fxp<+/-,24,5>, "offset"=w119:fxp<+/-,24,5>)
      n98 = Subtract(x=w276, y=w269) -> (x-y=→"AI0":dbl)
      n99 = Multiply(x=w231, y=w114) -> (x*y=w232:fxp<+/-,48,10>)
      n100 = Subtract(x=w271, y=w269) -> (x-y=→"AI1":dbl)
      n101 = Multiply(x=w230, y=w111) -> (x*y=w233:fxp<+/-,48,10>)
      n102 = Multiply(x=w133, y=w123) -> (x*y=w134:fxp<+/-,48,10>)
      n103 = Add(x=w283, y=w251) -> (x+y=w163:dbl)
      "Exhaust_T" <- w163
      n104 = Add(x=w279, y=w251) -> (x+y=w161:dbl)
      "Oil_T" <- w161
      n105 = Add(x=w253, y=w251) -> (x+y=w204:dbl)
      "Basement_T" <- w204
      n106 = Add(x=w235, y=w107) -> (x+y=w188:fxp<+/-,48,10>)
      "Exhaust_P" <- w188
      n107 = Add(x=w236, y=w104) -> (x+y=w190:fxp<+/-,48,10>)
      "Oil_P" <- w190
      n108 = Add(x=w281, y=w251) -> (x+y=w165:dbl)
      "Intercooler_In_T" <- w165
      n109 = Add(x=w280, y=w251) -> (x+y=w99:dbl)
      "Intercooler_Out_T" <- w99
      n110 = Add(x=w260, y=w251) -> (x+y=w158:dbl)
      "Coolant_Inlet_T" <- w158
      n111 = Add(x=w278, y=w251) -> (x+y=w154:dbl)
      "Coolant_Outlet_T" <- w154
      n112 = Divide(x=w241, y=60000.0) -> (x/y=w103:dbl)
      "Power" <- w103
      n113 = Multiply(x=w138, y=w117) -> (x*y=w137:fxp<+/-,48,10>)
      n114 = Multiply(x=w135, y=w120) -> (x*y=w136:fxp<+/-,48,10>)
      n115 = Greater?(x=w165, y="Intercooler_In_Temp_lim") -> (0:w132:bool)
      "Boolean" <- w132
      n116 = Greater?(x=w99, y="Intercooler_Out_Temp_lim") -> (0:w131:bool)
      "Boolean 7" <- w131
      n117 = Greater?(x=w158, y="Coolant_Inlet_Temp_Lim") -> (0:w199:bool)
      "Boolean 4" <- w199
      n118 = Greater?(x=w154, y="Coolant_Outlet_Temp_Lim") -> (0:w198:bool)
      "Boolean 5" <- w198
      n119 = Greater?(x=w204, y="Basement_Temp_Lim") -> (0:w197:bool)
      "Boolean 6" <- w197
      n120 = Add(x=w134, y=w122) -> (x+y=w92:fxp<+/-,48,10>)
      "Misc_P" <- w92
      n121 = Add(x=w232, y=w113) -> (x+y=w184:fxp<+/-,48,10>)
      "Coolant-In_P" <- w184
      n122 = Add(x=w233, y=w110) -> (x+y=w185:fxp<+/-,48,10>)
      "Coolant-Out_P" <- w185
      n123 = Subtract(x=w270, y=25.0) -> (x-y=→"AI2":dbl)
      n124 = Greater?(x=w161, y="Oil_Temp_Max_Lim") -> (0:w247:bool)
      n125 = Less?(x=w161, y="Oil_Temp_min_Lim") -> (x < y?=w246:bool)
      n126 = Subtract(x=w184, y="Ambient_pressure") -> (x-y=w182:fxp<+/-,49,11>)
      n127 = Subtract(x=w185, y="Ambient_pressure") -> (x-y=w186:fxp<+/-,49,11>)
      n128 = Subtract(x=w188, y="Ambient_pressure") -> (x-y=w187:fxp<+/-,49,11>)
      n129 = Greater?(x=w163, y="Exhaust_Temp_Lim") -> (0:w201:bool)
      "Boolean 2" <- w201
      n130 = Subtract(x=w190, y="Ambient_pressure") -> (x-y=w189:fxp<+/-,49,11>)
      n131 = Add(x=w137, y=w116) -> (x+y=w96:fxp<+/-,48,10>)
      "Intercooler-In_P" <- w96
      n132 = Add(x=w136, y=w119) -> (x+y=w94:fxp<+/-,48,10>)
      "Intercooler-Out_P" <- w94
      n133 = Get Date/Time In Seconds() -> (seconds since 1Jan1904=w175:timestamp)
      n134 = Greater?(x=w103, y="Power_Max_Lim") -> (0:w101:bool)
      n135 = Greater?(x=w182, y="Coolant In Pres_Lim") -> (0:w196:bool)
      n136 = Greater?(x=w186, y="CoolantOut_press_Lim") -> (0:w195:bool)
      n137 = Greater?(x=w187, y="Exhaust_Pres_Lim") -> (0:w194:bool)
      n138 = Greater?(x=w189, y="Oil_Pres_Max_lim") -> (0:w193:bool)
      n139 = Less?(x=w189, y="Oil_Pres_Min_lim") -> (x < y?=w192:bool)
      n140 = Greater?(x=w96, y="Intercooler-In_P_Lim") -> (0:w129:bool)
      n141 = Greater?(x=w94, y="Intercooler-Out_P_Lim") -> (0:w127:bool)
      n142 = Greater?(x=w92, y="Misc_P_Lim") -> (0:w125:bool)
      n143 = Format Date/Time String(time format string (%c)="%Y%m%d_%H%M%S", seconds (now)=w175) -> (date/time string=w174:string)  [unwired: 1 in]
      n144 = Or(x=w247, y=w246) -> (x .or. y?=w200:bool)
      "Boolean 3" <- w200
      n145 = Number To Fractional String(number=w170, precision (6)=i16 2) -> (F-format string=w221:string)  [unwired: 2 in]
      n146 = Number To Fractional String(number=w168, precision (6)=i16 2) -> (F-format string=w173:string)  [unwired: 2 in]
      n147 = Number To Fractional String(number=w146, precision (6)=i16 2) -> (F-format string=w219:string)  [unwired: 2 in]
      n148 = Number To Fractional String(number=w167, precision (6)=i16 2) -> (F-format string=w217:string)  [unwired: 2 in]
      n149 = Number To Fractional String(number=w142, precision (6)=i16 2) -> (F-format string=w218:string)  [unwired: 2 in]
      n150 = Number To Fractional String(number=w103, precision (6)=i16 2) -> (F-format string=w166:string)  [unwired: 2 in]
      n151 = Number To Fractional String(number=w165, precision (6)=i16 2) -> (F-format string=w164:string)  [unwired: 2 in]
      n152 = Number To Fractional String(number=w163, precision (6)=i16 2) -> (F-format string=w162:string)  [unwired: 2 in]
      n153 = Number To Fractional String(number=w161, precision (6)=i16 2) -> (F-format string=w159:string)  [unwired: 2 in]
      n154 = Number To Fractional String(number=w158, precision (6)=i16 2) -> (F-format string=w157:string)  [unwired: 2 in]
      n155 = Number To Fractional String(number=w154, precision (6)=i16 2) -> (F-format string=w153:string)  [unwired: 2 in]
      n156 = Number To Fractional String(number=w184, precision (6)=i16 2) -> (F-format string=w152:string)  [unwired: 2 in]
      n157 = Number To Fractional String(number=w185, precision (6)=i16 2) -> (F-format string=w151:string)  [unwired: 2 in]
      n158 = Number To Fractional String(number=w188, precision (6)=i16 2) -> (F-format string=w150:string)  [unwired: 2 in]
      n159 = Number To Fractional String(number=w190, precision (6)=i16 2) -> (F-format string=w149:string)  [unwired: 2 in]
      n160 = Number To Fractional String(number=w99, precision (6)=i16 2) -> (F-format string=w98:string)  [unwired: 2 in]
      n161 = Number To Fractional String(number=w96, precision (6)=i16 2) -> (F-format string=w91:string)  [unwired: 2 in]
      n162 = Number To Fractional String(number=w94, precision (6)=i16 2) -> (F-format string=w90:string)  [unwired: 2 in]
      n163 = Number To Fractional String(number=w92, precision (6)=i16 2) -> (F-format string=w89:string)  [unwired: 2 in]
      n164 = Build Array(w174, w221, w173, w219, w217, w218, w166, w164, w162, w159, w157, w153, w152, w151, w150, w149, w98, w91, w90, w89, w77, w76, w75, w74) -> (w229:string[])
      n165 = And(x=w192, y=w179) -> (x .and. y?=w180:bool)
      n166 = Compound Arithmetic op=OR(w101, w132, w131, w201, w200, w199, w198, w197, w196, w195, w194, w193, w180, w144, w143, w140, w129, w127, w125) -> (w191:bool)
      "Saftey_Lim_error" <- w191
      n167 = case shown="True" "Data_Log" {
        tunnel: w229 -> [_ w314]
        tunnel: w227 -> [_ w318]
        tunnel: w226 -> [w313 w317]
        tunnel: [w313 w316] -> w225
        frame False {
        }
        frame True {
          n168 = call-poly <vilib>:"Write Delimited Spreadsheet.vi"("file path (dialog if empty)"=w317, "1D data"=w314, "append to file? (new file:F)"=TRUE, "error in (no error)"=w318, "delimiter (\\t)"="," ("delimiter (\\t)")) -> ("new file path (Not A Path if cancelled)"=w316:path)  [unwired: 9 in, 1 out]
        }
      }
      n169 = Build Array(w191) -> (w148:bool[])
      n170 = shared-variable "My Computer\\test_1.lvlib\\Data_Bool"(w148) -> ()  [unwired: 1 in, 1 out]
      n171 = local read "Stop"() -> (w282:bool)
    }
    n172 = while {
      tunnel: w60 -> [w335]
      tunnel: w59 -> [w334]
      tunnel: [w333] -> w58
      tunnel: [w332] -> w57
      stop <- w331 stop-if-true
      w320 = 10.0 ("y")
      n173 = local read "Coolant_Outlet_T"() -> (w325:dbl)
      n174 = Divide(x=w325, y=w320) -> (x/y=w321:dbl)
      n175 = Divide(x="Temperature", y=w320) -> (x/y=w324:dbl)
      n176 = call-poly <vilib>:"PID.vi"("output range"="Output range", "dt (s)"=-1.0, "PID gains"="PID gains", "process variable"=w321, "setpoint"=w324) -> ("output"=w328:dbl)  [unwired: 5 in, 1 out]
      n177 = Select(t=w328, s="Temperature PID", f=w324) -> (s? t:f=w323:dbl)
      "Temperature out" <- w323
      n178 = xnode "Read/Write Control"("FPGA VI Reference In"=w335, "error in"=w334, "Cooling  Set point (°C)"=w323) -> ("FPGA VI Reference Out"=w333:refnum<k20>, "error out"=w332:errorcluster)
      n179 = local read "Stop"() -> (w331:bool)
    }
    n180 = xnode "Invoke Method"("FPGA VI Reference In"=w58, "error in"=w57) -> ("FPGA VI Reference Out"=w56:refnum<k20>, "error out"=w55:errorcluster)
    n181 = xnode "Close FPGA VI Reference"("FPGA VI Reference In"=w56, "error in"=w55) -> ()  [unwired: 1 out]
    n182 = xnode "Invoke Method"("FPGA VI Reference In"=w51, "error in"=w50) -> ("FPGA VI Reference Out"=w67:refnum<k20>, "error out"=w66:errorcluster)
    n183 = xnode "Close FPGA VI Reference"("FPGA VI Reference In"=w67, "error in"=w66) -> ()  [unwired: 1 out]
  }
  n184 = call <vilib>:"Add State(s) to Queue__JKI_lib_State_Machine.vi"("State(s) in (\"\")"="Macro: Initialize") -> ("States Out"=w3:string)  [unwired: 14 in]
  n185 = while "JKI State Machine 2018" {
    shift-right: [w339] -> _
    shift-left: _ -> [w338]
    shift-right: [w342] -> _
    shift-left: errorcluster {"status"=FALSE, "code"=0, "source"=""} ("error out") -> [w336]
    shift-right: [w341] -> _
    shift-left: w3 -> [w343]
    stop <- w340 stop-if-true
    w337 = -1  # Timeout
    n186 = call <vilib>:"Parse State Queue__JKI_lib_State_Machine.vi"("State Queue"=w343, "Error In (no error)"=w336) -> ("Remaining States"=w345:string, "Current State"=w346:string, "Arguments"=w344:string)  [unwired: 11 in]
    n187 = case shown="\"Exit\"" w346 {
      selector: w346 -> [_ _ w373 _ _ _ _ _ _ _ _ _ _ _ _ _ _ _ _]
      tunnel: w345 -> [w353 w372 w377 w396 w402 w407 w411 w424 w430 w434 w443 w528 w534 w545 w614 w619 w629 w633 w637]
      tunnel: w344 -> [_ _ _ _ _ _ _ _ _ _ _ _ w529 w539 _ _ _ _ _]
      tunnel: w338 -> [w351 w369 w375 w389 w399 w405 w408 _ w425 w431 w440 w526 w532 w541 w611 w616 w626 w630 w634]
      tunnel: [w350 w370 w379 w393 errorcluster {"status"=FALSE, "code"=0, "source"=""} ("error out") w404 w409 w421 w426 w432 w435 w449 w530 w542 w612 w617 w627 w631 w635] -> w342
      tunnel: w336 -> [w349 w370 w378 w393 w398 w404 w409 w421 w427 w432 w437 w520 w531 w543 w612 w617 w627 w631 w635]
      tunnel: [w352 w371 w376 w395 w401 w406 w410 w423 w429 w433 w442 w527 w533 w544 w613 w618 w628 w632 w636] -> w341
      tunnel: [_ _ _ _ _ TRUE _ _ _ _ _ _ _ _ _ _ _ _ _] -> w340
      tunnel: [w348 w369 w375 w394 w399 w405 w408 w422 w425 w431 w440 w526 w532 w541 w611 w616 w626 w630 w634] -> w339
      tunnel: w337 -> [w347 _ _ _ _ _ _ _ _ _ _ _ _ _ _ _ _ _ _]
      frame "", "Event Structure", "Idle" {
        # "executes when the state queue is empty"
        n188 = event shown="[2] Panel Close?" {
          selector: _ -> [_ _ _]
          dyn-events: _ -> [_ _ _]
          timeout: w347 -> [_ _ _]
          tunnel: w353 -> [w357 w362 w368]
          tunnel: [w356 w361 w367] -> w352
          tunnel: w351 -> [w354 w359 w365]
          tunnel: [w355 w360 w366] -> w350
          tunnel: w349 -> [w355 w360 w366]
          tunnel: [w354 w359 w365] -> w348
          event Timeout {
            n189 = event-data() -> ()  [unwired: 1 in, 1 out]
            n190 = call <vilib>:"Add State(s) to Queue__JKI_lib_State_Machine.vi"("State(s) in (\"\")"=w357) -> ("States Out"=w356:string)  [unwired: 14 in]
          }
          event "Stop": Value Change {
            # "Exit Button Value Change (pressed) Event\n(this executes Macro: Exit to terminate the VI)"
            n191 = event-data() -> ()  [unwired: 1 in, 6 out]
            n192 = call <vilib>:"Add State(s) to Queue__JKI_lib_State_Machine.vi"("State(s) in Front (\"\")"="Macro: Exit", "State(s) in (\"\")"=w362) -> ("States Out"=w361:string)  [unwired: 13 in]
          }
          event Panel Close? {
            # "Discard the event because we'll close the front panel ourselves in Macro: Exit"
            # "Close Panel button (pressed) Event\n(this executes Macro: Exit to terminate the VI)"
            n193 = event-data() -> ()  [unwired: 1 in, 1 out]
            n194 = event-data("Discard?"=TRUE) -> ()  [unwired: 1 in, 1 out]
            n195 = call <vilib>:"Add State(s) to Queue__JKI_lib_State_Machine.vi"("State(s) in Front (\"\")"="Macro: Exit", "State(s) in (\"\")"=w368) -> ("States Out"=w367:string)  [unwired: 13 in]
          }
        }
      }
      frame "---------- Core ----------" {
        # "Do not put any code in this frame.\n(it is a separator no-op)"
        n196 = call <vilib>:"Add State(s) to Queue__JKI_lib_State_Machine.vi"("State(s) in (\"\")"=w372) -> ("States Out"=w371:string)  [unwired: 14 in]
      }
      frame Default {
        w382 = 42 items=["No error", "Argument error", "Memory is full", "Out of zone", "End of file", "File already open", "Generic file I/O error", "File not found", "File permission error", "Disk is full", "Duplicate path", "Too many files open", "System feature not enabled", "Resource file not found", "Cannot add resource", "Resource not found", "Image not found", "Image memory error", "Pen does not exist", "Config type invalid", "Config token not found", "Config parse error", "Config memory error", "Bad external code format", "Bad external code offset", "External code not present", "Null window", "Destroy window error", "Null menu", "Print aborted", "Bad print record", "Print driver error", "Windows error during printing", "Memory error during printing", "Print dialog error", "Generic print error", "Invalid device refnum", "Device not found", "Device parameter error", "Device unit error", "Cannot open device", "Device call aborted", "Generic error", "Cancelled by user", "Object ID too low", "Object ID too high", "Object not in heap", "Unknown heap", "Unknown object (invalid DefProc)", "Unknown object (DefProc not in table)", "Message out of range", "Invalid (null) method", "Unknown message", "Manager call not supported", "Bad address", "Network operation in progress", "Network operation timed out", "Connection is busy", "Network attribute not supported", "Network error", "Address in use", "System out of memory", "Connection aborted", "Connection refused", "Not connected", "Already connected", "Connection closed", "Initialization error (interapplication manager)", "Bad occurrence", "Wait on unbound occurrence handler", "Occurrence queue overflow", "Datalog type conflict", "Unused", "Unrecognized type (interapplication manager)", "Memory corrupt", "Failed to make temporary DLL", "Old CIN version", "Drag socket not found", "Failed to load drop-object", "Failed to register OLE object", "Failed to release OLE object", "Format specifier type mismatch", "Unknown format specifier", "Too few format specifiers", "Too many format specifiers", "Scan failed", "Newer CIN version", "Error converting to variant", "Runtime menu error", "Password tampered", "Variant attribute not found", "Incompatible variant data type", "Event data is not available", "Event Store is not present", "Occurrence is not found", "Event Queue is not created", "Event info is not available", "Refnum passed is NULL", "Error retrieving Class GUID", "Error retrieving CoClass GUID", "Error retrieving TypeLib GUID.", "Bad built application magic bytes.", "Specific driver is different from the specific driver associated with the Logical Name.", "There is no session opened to the class driver.", "Max Error", "MAX - Error with config objects", "MAX - Error loading configuration", "MAX - Group not supported"]
        # "Current State"
        # "Do not delete, rename, or modify this frame.\n(this is used to capture unhandled states and typos)"
        # "Handle mistyped state name (developer tool)"
        n197 = Format Into String(format string="Software Exception: Unhandled State \"%s\"." ("message"), error in=w378, w373) -> (resulting string=w381:string, error out=w380:errorcluster)  [unwired: 1 in]
        n198 = call <vilib>:"Error Cluster From Error Code.vi"("show call chain? (False)"=TRUE, "error in (no error)"=w380, "error message (\"\")"=w381, "error code (0)"=w382) -> ("error out"=w379:errorcluster)  [unwired: 5 in]
        n199 = call <vilib>:"Add State(s) to Queue__JKI_lib_State_Machine.vi"("State(s) in (\"\")"=w377) -> ("States Out"=w376:string)  [unwired: 14 in]
      }
      frame "Initialize Core Data" {
        # "Do not delete, rename, or modify this frame.\n(this is used to determine panel behavior on exit)"
        # "originally closed?"
        # "exe?"
        # "If panel starts closed or is an EXE, then close it when we exit"
        n200 = property class="VI"() -> ("FP.State"=w386:T3)  [unwired: 2 in, 2 out]
        n201 = property class="App"() -> ("App.Kind"=w392:T4)  [unwired: 2 in, 2 out]
        n202 = control-ref of="Current VI Reference"() -> (w387:refnum<vi>)
        n203 = Equal?(x=w386, y=T3."Closed" ("Front Panel Window:State")) -> (x = y?=w384:bool)
        n204 = Equal?(x=w392, y=T4."Run Time System" ("Application:Kind")) -> (x = y?=w390:bool)
        n205 = Or(x=w384, y=w390) -> (x .or. y?=w388:bool)
        n206 = Bundle By Name(cluster=w389, "Core.Current VI Reference"=w387, "Core.Close Panel on Exit?"=w388) -> (w394:T5)
        n207 = call <vilib>:"Add State(s) to Queue__JKI_lib_State_Machine.vi"("State(s) in (\"\")"=w396) -> ("States Out"=w395:string)  [unwired: 14 in]
      }
      frame "Error Handler" {
        # "Unhandled Error -- Display it"
        # "Handle any errors here.\nYou can also output any states to clean-up after errors occur"
        # "Clear error"
        n208 = call <vilib>:"General Error Handler.vi"("error in (no error)"=w398) -> ()  [unwired: 10 in, 5 out]
        n209 = call <vilib>:"Add State(s) to Queue__JKI_lib_State_Machine.vi"("State(s) in Front (\"\")"="/* Post Error States", "State(s) in (\"\")"=w402) -> ("States Out"=w401:string)  [unwired: 13 in]
      }
      frame "Exit" {
        # "Do not put any code in this frame.\n(No errors that occur here will be handled.)"
        n210 = call <vilib>:"Add State(s) to Queue__JKI_lib_State_Machine.vi"("State(s) in (\"\")"=w407) -> ("States Out"=w406:string)  [unwired: 14 in]
      }
      frame "---------- Data ----------" {
        # "Do not put any code in this frame.\n(It is a separator no-op. You can make a copy of this frame to create a new Data frame)"
        n211 = call <vilib>:"Add State(s) to Queue__JKI_lib_State_Machine.vi"("State(s) in (\"\")"=w411) -> ("States Out"=w410:string)  [unwired: 14 in]
      }
      frame "Data: Initialize" {
        w412 = refnum<k20> refnum  # ExpansionChassFPGA
        w420 = T6 {"Current VI Reference"=refnum, "Close Panel on Exit?"=FALSE}  # Core
        # "Initialize the shift-register data, here.\n(data names are defined by what you wire into the bundle function)"
        n212 = control-ref of="Intercooler_In_T"() -> (w419:refnum<vi>)
        n213 = control-ref of="Coolant_Inlet_T"() -> (w418:refnum<vi>)
        n214 = control-ref of="Coolant_Outlet_T"() -> (w417:refnum<vi>)
        n215 = control-ref of="Basement_T"() -> (w416:refnum<vi>)
        n216 = control-ref of="Exhaust_T"() -> (w415:refnum<vi>)
        n217 = control-ref of="Oil_T"() -> (w414:refnum<vi>)
        n218 = control-ref of="Intercooler_Out_T"() -> (w413:refnum<vi>)
        n219 = Bundle("Core"=w420, "Intercooler_In_T"=w419, "Coolant_Inlet_T"=w418, "Coolant_Outlet_T"=w417, "Basement_T"=w416, "Exhaust_T"=w415, "Oil_T"=w414, "Intercooler_Out_T"=w413, "ExpansionChassFPGA"=w412) -> (w422:T5)  [unwired: 1 in]
        n220 = call <vilib>:"Add State(s) to Queue__JKI_lib_State_Machine.vi"("State(s) in (\"\")"=w424) -> ("States Out"=w423:string)  [unwired: 14 in]
      }
      frame "Data: Cleanup" {
        # "Cleanup any data and references, here.\n(this is called automatically, by the Macro: Exit)"
        n221 = Unbundle By Name(w425) -> ("Core.Current VI Reference"=w428:refnum<vi>)
        n222 = Close Reference(reference=w428, error in (no error)=w427) -> (error out=w426:errorcluster)
        n223 = call <vilib>:"Add State(s) to Queue__JKI_lib_State_Machine.vi"("State(s) in (\"\")"=w430) -> ("States Out"=w429:string)  [unwired: 14 in]
      }
      frame "---------- UI ----------" {
        # "Do not put any code in this frame.\n(It is a separator no-op. You can make a copy of this frame to create a new UI frame)"
        n224 = call <vilib>:"Add State(s) to Queue__JKI_lib_State_Machine.vi"("State(s) in (\"\")"=w434) -> ("States Out"=w433:string)  [unwired: 14 in]
      }
      frame "UI: Initialize" {
        # "Initialize the User Interface, here.\n(this is called automatically, by the Macro: Init)"
        n225 = Unbundle By Name(w440) -> ("Core.Current VI Reference"=w439:refnum<vi>)
        n226 = property class="VI"(reference=w439, error in=w437, "FP.Monitor"=u16 2 ("Front Panel Window:Monitor")) -> (error out=w436:errorcluster)  [unwired: 1 out]
        n227 = call <vilib>:"Clear Errors.vi"("error in (no error)"=w436) -> ("error out"=w435:errorcluster)  [unwired: 5 in, 1 out]
        n228 = call <vilib>:"Add State(s) to Queue__JKI_lib_State_Machine.vi"("State(s) in (\"\")"=w443, "State(s) at Back (\"\")"="Set Scale.Marker" ("State(s) at Back (\"\")")) -> ("States Out"=w442:string)  [unwired: 13 in]
      }
      frame "Set Scale.Marker" {
        n229 = Unbundle By Name(w526) -> ("Intercooler_Out_T"=w450:refnum<vi>, "Coolant_Inlet_T"=w525:refnum<vi>, "Coolant_Outlet_T"=w524:refnum<vi>, "Basement_T"=w523:refnum<vi>, "Exhaust_T"=w522:refnum<vi>, "Oil_T"=w521:refnum<vi>)  [unwired: 1 out]
        n230 = Bundle(60.0, u32 16776002) -> (w518:cluster{dbl, u32})  [unwired: 1 in]
        n231 = Bundle(70.0, u32 16711680) -> (w517:cluster{dbl, u32})  [unwired: 1 in]
        n232 = Bundle(100.0, u32 0) -> (w516:cluster{dbl, u32})  [unwired: 1 in]
        n233 = Bundle(40.0, u32 16776002) -> (w490:cluster{dbl, u32})  [unwired: 1 in]
        n234 = Bundle(50.0, u32 16711680) -> (w491:cluster{dbl, u32})  [unwired: 1 in]
        n235 = Bundle(60.0, u32 0) -> (w492:cluster{dbl, u32})  [unwired: 1 in]
        n236 = Bundle(70.0, u32 2027264) -> (w507:cluster{dbl, u32})  [unwired: 1 in]
        n237 = Bundle(90.0, u32 16776002) -> (w506:cluster{dbl, u32})  [unwired: 1 in]
        n238 = Bundle(100.0, u32 16711680) -> (w505:cluster{dbl, u32})  [unwired: 1 in]
        n239 = Bundle(120.0, u32 0) -> (w504:cluster{dbl, u32})  [unwired: 1 in]
        n240 = Bundle(0.0, u32 2027264) -> (w519:cluster{dbl, u32})  [unwired: 1 in]
        n241 = Bundle(0.0, u32 2027264) -> (w489:cluster{dbl, u32})  [unwired: 1 in]
        n242 = Bundle(0.0, u32 16776002) -> (w503:cluster{dbl, u32})  [unwired: 1 in]
        n243 = Build Array(w519, w518, w517, w516) -> (w448:cluster{dbl, u32}[])
        n244 = Build Array(w489, w490, w491, w492) -> (w446:cluster{dbl, u32}[])
        n245 = Build Array(w503, w507, w506, w505, w504) -> (w447:cluster{dbl, u32}[])
        n246 = Build Array(w450, w525, w524, w523, w522, w521) -> ()  [unwired: 1 out]
        n247 = property on="Coolant_Inlet_T" class="Knob (strict)"("Scale.MarkerVals[]"=w447) -> ()  [unwired: 2 in, 2 out]
        n248 = property on="Coolant_Outlet_T" class="Knob (strict)"("Scale.MarkerVals[]"=w447) -> ()  [unwired: 2 in, 2 out]
        n249 = property on="Basement_T" class="Knob (strict)"("Scale.MarkerVals[]"=w446) -> ()  [unwired: 2 in, 2 out]
        n250 = property on="Intercooler_Out_T" class="Knob (strict)"("Scale.MarkerVals[]"=w448) -> ()  [unwired: 2 in, 2 out]
        n251 = property on="Intercooler_In_T" class="Knob (strict)"("Scale.MarkerVals[]"=w448) -> ()  [unwired: 2 in, 2 out]
        n252 = Bundle(800.0, u32 16776002) -> (w478:cluster{dbl, u32})  [unwired: 1 in]
        n253 = Bundle(900.0, u32 16711680) -> (w479:cluster{dbl, u32})  [unwired: 1 in]
        n254 = Bundle(1000.0, u32 0) -> (w480:cluster{dbl, u32})  [unwired: 1 in]
        n255 = Bundle(40.0, u32 16776002) -> (w467:cluster{dbl, u32})  [unwired: 1 in]
        n256 = Bundle(70.0, u32 6618880) -> (w466:cluster{dbl, u32})  [unwired: 1 in]
        n257 = Bundle(110.0, u32 16776002) -> (w465:cluster{dbl, u32})  [unwired: 1 in]
        n258 = Bundle(120.0, u32 16713728) -> (w464:cluster{dbl, u32})  [unwired: 1 in]
        n259 = Bundle(140.0, u32 0) -> (w463:cluster{dbl, u32})  [unwired: 1 in]
        n260 = Bundle(0.0, u32 2027264) -> (w477:cluster{dbl, u32})  [unwired: 1 in]
        n261 = call <vilib>:"Clear Errors.vi"("error in (no error)"=w520) -> ("error out"=w449:errorcluster)  [unwired: 5 in, 1 out]
        n262 = Bundle(0.0, u32 16713728) -> (w468:cluster{dbl, u32})  [unwired: 1 in]
        n263 = Build Array(w477, w478, w479, w480) -> (w445:cluster{dbl, u32}[])
        n264 = Build Array(w468, w467, w466, w465, w464, w463) -> (w444:cluster{dbl, u32}[])
        n265 = property on="Exhaust_T" class="Knob (strict)"("Scale.MarkerVals[]"=w445) -> ()  [unwired: 2 in, 2 out]
        n266 = property on="Oil_T" class="Knob (strict)"("Scale.MarkerVals[]"=w444) -> ()  [unwired: 2 in, 2 out]
        n267 = call <vilib>:"Add State(s) to Queue__JKI_lib_State_Machine.vi"("State(s) in (\"\")"=w528) -> ("States Out"=w527:string)  [unwired: 14 in]
      }
      frame "UI: Cursor Set" {
        # "Argument"
        # "Set and Unset Cursor Busy.\n(Usage: \"UI: Cursor Set >> Busy|Idle\")"
        n268 = case shown="\"Idle\", Default" w529 {
          tunnel: w531 -> [w536 w538]
          tunnel: [w535 w537] -> w530
          frame "Idle", Default {
            n269 = call <vilib>:"Unset Busy.vi"("error in (no error)"=w536) -> ("error out"=w535:errorcluster)  [unwired: 10 in]
          }
          frame "Busy" {
            n270 = call <vilib>:"Set Busy.vi"("error in (no error)"=w538) -> ("error out"=w537:errorcluster)  [unwired: 9 in, 1 out]
          }
        }
        n271 = call <vilib>:"Add State(s) to Queue__JKI_lib_State_Machine.vi"("State(s) in (\"\")"=w534) -> ("States Out"=w533:string)  [unwired: 14 in]
      }
      frame "UI: Front Panel State" {
        # "Argument"
        # "Set Front Panel Open or Closed\n(Usage: \"UI: Front Panel State >> Open|Close\")"
        n272 = Unbundle By Name(w541) -> ("Core.Current VI Reference"=w540:refnum<vi>)
        n273 = case shown="\"Minimize\", \"Minimized\"" w539 {
          tunnel: w543 -> [w551 w566 w577 w590 w603]
          tunnel: [w553 w567 w579 w592 w605] -> w542
          tunnel: w540 -> [w552 w564 w578 w591 w604]
          frame "Open", "Standard", Default {
            w546 = T3."Standard" ("State")
            n274 = property class="VI"(reference=w552, error in=w551) -> (reference out=w549:refnum<vi>, error out=w550:errorcluster, "FP.State"=w548:T3)
            n275 = Not Equal?(x=w548, y=w546) -> (x != y?=w547:bool)
            n276 = case shown="True" w547 {
              tunnel: [w557 w559] -> w553
              tunnel: w550 -> [w556 w559]
              tunnel: w549 -> [w555 _]
              tunnel: w546 -> [w554 _]
              frame True {
                n277 = invoke class="VI" method="FP.Open"(reference=w555, error in=w556, "Activate"=TRUE, "State"=w554) -> (error out=w557:errorcluster)  [unwired: 1 in, 4 out]
              }
              frame False {
              }
            }
          }
          frame "Close", "Closed" {
            n278 = property class="VI"(reference=w564, error in=w566) -> (reference out=w563:refnum<vi>, error out=w565:errorcluster, "FP.State"=w561:T3)
            n279 = Not Equal?(x=w561, y=T3."Closed" ("Front Panel Window:State")) -> (x != y?=w560:bool)
            n280 = case shown="True" w560 {
              tunnel: [w568 w571] -> w567
              tunnel: w565 -> [w568 w570]
              tunnel: w563 -> [_ w569]
              frame False {
              }
              frame True {
                n281 = invoke class="VI" method="FP.Close"(reference=w569, error in=w570) -> (error out=w571:errorcluster)  [unwired: 1 in, 2 out]
              }
            }
          }
          frame "Hidden", "Hide" {
            w572 = T3."Hidden" ("State")
            n282 = property class="VI"(reference=w578, error in=w577) -> (reference out=w575:refnum<vi>, error out=w576:errorcluster, "FP.State"=w574:T3)
            n283 = Not Equal?(x=w574, y=w572) -> (x != y?=w573:bool)
            n284 = case shown="True" w573 {
              tunnel: [w583 w584] -> w579
              tunnel: w576 -> [w582 w584]
              tunnel: w575 -> [w581 _]
              tunnel: w572 -> [w580 _]
              frame True {
                n285 = invoke class="VI" method="FP.Open"(reference=w581, error in=w582, "State"=w580) -> (error out=w583:errorcluster)  [unwired: 2 in, 4 out]
              }
              frame False {
              }
            }
          }
          frame "Minimize", "Minimized" {
            w585 = T3."Minimized" ("State")
            n286 = property class="VI"(reference=w591, error in=w590) -> (reference out=w588:refnum<vi>, error out=w589:errorcluster, "FP.State"=w587:T3)
            n287 = Not Equal?(x=w587, y=w585) -> (x != y?=w586:bool)
            n288 = case shown="False" w586 {
              tunnel: [w596 w597] -> w592
              tunnel: w589 -> [w595 w597]
              tunnel: w588 -> [w594 _]
              tunnel: w585 -> [w593 _]
              frame True {
                n289 = invoke class="VI" method="FP.Open"(reference=w594, error in=w595, "State"=w593) -> (error out=w596:errorcluster)  [unwired: 2 in, 4 out]
              }
              frame False {
              }
            }
          }
          frame "Maximize", "Maximized" {
            w598 = T3."Maximized" ("State")
            n290 = property class="VI"(reference=w604, error in=w603) -> (reference out=w601:refnum<vi>, error out=w602:errorcluster, "FP.State"=w600:T3)
            n291 = Not Equal?(x=w600, y=w598) -> (x != y?=w599:bool)
            n292 = case shown="True" w599 {
              tunnel: [w609 w610] -> w605
              tunnel: w602 -> [w608 w610]
              tunnel: w601 -> [w607 _]
              tunnel: w598 -> [w606 _]
              frame True {
                n293 = invoke class="VI" method="FP.Open"(reference=w607, error in=w608, "State"=w606) -> (error out=w609:errorcluster)  [unwired: 2 in, 4 out]
              }
              frame False {
              }
            }
          }
        }
        n294 = call <vilib>:"Add State(s) to Queue__JKI_lib_State_Machine.vi"("State(s) in (\"\")"=w545) -> ("States Out"=w544:string)  [unwired: 14 in]
      }
      frame "---------- Macro ----------" {
        # "Do not put any code in this frame.\n(It is a separator no-op. You can make a copy of this frame to create a new Macro frame)"
        n295 = call <vilib>:"Add State(s) to Queue__JKI_lib_State_Machine.vi"("State(s) in (\"\")"=w614) -> ("States Out"=w613:string)  [unwired: 14 in]
      }
      frame "Macro: Initialize" {
        w615 = "Data: Initialize\nInitialize Core Data\nUI: Initialize\nUI: Front Panel State >> Open"  # Data: Initialize Initialize Core Data UI: Initialize UI: Front Panel State >> Open
        # "Initialization Macro\n(This is called once, when the VI starts)"
        n296 = call <vilib>:"Add State(s) to Queue__JKI_lib_State_Machine.vi"("State(s) in Front (\"\")"=w615, "State(s) in (\"\")"=w619) -> ("States Out"=w618:string)  [unwired: 13 in]
      }
      frame "Macro: Exit" {
        # "Exit Macro\n(This is called once, when the VI exits)"
        n297 = Unbundle By Name(w626) -> ("Core.Close Panel on Exit?"=w625:bool)
        n298 = Select(t="UI: Front Panel State >> Close", s=w625, f="") -> (s? t:f=w622:string)
        n299 = call <vilib>:"Add State(s) to Queue__JKI_lib_State_Machine.vi"("State(s) in (\"\")"=w622, "State(s) at Back (\"\")"="Data: Cleanup\nExit") -> ("States Out"=w620:string)  [unwired: 13 in]
        n300 = call <vilib>:"Add State(s) to Queue__JKI_lib_State_Machine.vi"("State(s) in Front (\"\")"=w620, "State(s) in (\"\")"=w629) -> ("States Out"=w628:string)  [unwired: 13 in]
      }
      frame "---------- New Category ----------" {
        # "Template Separator\n(You can make a copy of, or modify, this frame)"
        n301 = call <vilib>:"Add State(s) to Queue__JKI_lib_State_Machine.vi"("State(s) in (\"\")"=w633) -> ("States Out"=w632:string)  [unwired: 14 in]
      }
      frame "New Category: 2" {
        # "Your code here.\n(You can make a copy of, or modify, this frame)"
        n302 = call <vilib>:"Add State(s) to Queue__JKI_lib_State_Machine.vi"("State(s) in (\"\")"=w637) -> ("States Out"=w636:string)  [unwired: 14 in]
      }
    }
  }
